vi "BRig_RT_panel_Laser2_v1,10.vi"(7 "input_setValues":bool, 9 "input_dataExp":u16[](array[numeric]), 11 "input_dataLC":u16[](array[numeric])) -> (1 "output_dataExp":u16[](array[numeric]), 3 "output_dataLC":u16[](array[numeric]))   [LabVIEW 2014]
panel:
  in  "LC_Cue2_PostR_Count":u16
  in  "LC_Cue2_PostR_delayOpt":bool
  in  "LC_Cue2_PostR_Probability":u16
  in  "LC_Cue2_PostR_Block":u16(slide) max=2 step=1 scale=0.0..2.0
  in  "LC_Cue2_PostR_OnOff":bool
  in  "LC_Cue2_PostR_Tdelay":u16
  in  "LC_ENL2_PostR_delayOpt":bool
  in  "LC_ENL2_PostR_Count":u16
  in  "LC_ENL2_PostR_Probability":u16 max=100 step=1
  in  "LC_ENL2_PostR_Block":u16(slide) max=2 step=1 scale=0.0..2.0
  in  "LC_ENL2_PostR_OnOff":bool
  in  "LC_ENL2_PostR_Tdelay":u16
  in  "LC_Cue2_PreR_Count":u16
  in  "LC_Cue2_First_Count":u16
  in  "LC_Cue2_PreR_delayOpt":bool
  in  "LC_ENL2_PreR_delayOpt":bool
  in  "LC_ENL2_PreR_Count":u16
  in  "LC_ENL2_First_Count":u16
  in  "LC_Cue2_First_delayOpt":bool
  in  "LC_ENL2_First_delayOpt":bool
  in  "LC_Cue2_PreR_Probability":u16
  in  "LC_Cue2_PreR_Block":u16(slide) max=2 step=1 scale=0.0..2.0
  in  "LC_Cue2_PreR_OnOff":bool
  in  "LC_Cue2_First_Probability":u16
  in  "LC_Cue2_First_Block":u16(slide) max=2 step=1 scale=0.0..2.0
  in  "LC_Cue2_First_OnOff":bool
  in  "LC_ENL2_PreR_Probability":u16 max=100 step=1
  in  "LC_ENL2_PreR_Block":u16(slide) max=2 step=1 scale=0.0..2.0
  in  "LC_ENL2_PreR_OnOff":bool
  in  "LC_ENL2_First_Probability":u16 max=100 step=1
  in  "LC_ENL2_First_Block":u16(slide) max=2 step=1 scale=0.0..2.0
  in  "LC_Cue2_PreR_Tdelay":u16
  in  "LC_ENL2_PreR_Tdelay":u16
  in  "LC_Cue2_First_Tdelay":u16
  in  "LC_ENL2_First_Tdelay":u16
  in  "LC_ENL2_First_OnOff":bool
  out "LaserPulseTrain":cluster{u16[], u16[]}(graph)
  in  "LED_baseline":bool
  in  "Laser_power_step":dbl
  in  "Laser_power_max":dbl
  in  "Laser_power_min":dbl
  in  "Laser_Tshutter":u16=2
  in  "Laser_Freq":u16=10
  in  "Laser_Tpeak":u16=2
  in  "Laser_T":u16
  in  "LC_Sel_PostR_Count":u16
  in  "LC_Sel_PostR_Probability":u16
  in  "LC_Sel_PostR_Block":u16(slide) max=2 step=1 scale=0.0..2.0
  in  "LC_Sel_PostR_OnOff":bool
  in  "LC_Sel_PostR_Tdelay":u16
  in  "LC_Cue_PostR_Count":u16
  in  "LC_Cue_PostR_delayOpt":bool
  in  "LC_Cue_PostR_Probability":u16
  in  "LC_Cue_PostR_Block":u16(slide) max=2 step=1 scale=0.0..2.0
  in  "LC_Cue_PostR_OnOff":bool
  in  "LC_Cue_PostR_Tdelay":u16
  in  "LC_ENL_PostR_delayOpt":bool
  in  "LC_ENL_PostR_Count":u16
  in  "LC_ENL_PostR_Probability":u16 max=100 step=1
  in  "LC_ENL_PostR_Block":u16(slide) max=2 step=1 scale=0.0..2.0
  in  "LC_ENL_PostR_OnOff":bool
  in  "LC_ENL_PostR_Tdelay":u16
  in  "LC_Sel_PreR_Count":u16
  in  "LC_Sel_First_Count":u16
  in  "LC_Sel_PreR_Probability":u16
  in  "LC_Sel_PreR_Block":u16(slide) max=2 step=1 scale=0.0..2.0
  in  "LC_Sel_PreR_OnOff":bool
  in  "LC_Sel_First_Probability":u16
  in  "LC_Sel_First_Block":u16(slide) max=2 step=1 scale=0.0..2.0
  in  "LC_Sel_First_OnOff":bool
  in  "LC_Sel_PreR_Tdelay":u16
  in  "LC_Sel_First_Tdelay":u16
  in  "LC_Cue_PreR_Count":u16
  in  "LC_Cue_First_Count":u16
  in  "LC_Cue_PreR_delayOpt":bool
  in  "LC_ENL_PreR_delayOpt":bool
  in  "LC_ENL_PreR_Count":u16
  in  "LC_ENL_First_Count":u16
  in  "LC_Cue_First_delayOpt":bool
  in  "LC_ENL_First_delayOpt":bool
  in  "LC_Wrong_Probability":u16
  in  "LC_Wrong_Trial":u16(slide) max=2 step=1 scale=0.0..2.0
  in  "LC_Wrong_Block":u16(slide) max=2 step=1 scale=0.0..2.0
  in  "LC_Wrong_OnOff":bool
  in  "LC_Reward_Probability":u16
  in  "LC_Reward_Trial":u16(slide) max=2 step=1 scale=0.0..2.0
  in  "LC_Reward_Block":u16(slide) max=2 step=1 scale=0.0..2.0
  in  "LC_Reward_OnOff":bool
  in  "LC_Cue_PreR_Probability":u16
  in  "LC_Cue_PreR_Block":u16(slide) max=2 step=1 scale=0.0..2.0
  in  "LC_Cue_PreR_OnOff":bool
  in  "LC_Cue_First_Probability":u16
  in  "LC_Cue_First_Block":u16(slide) max=2 step=1 scale=0.0..2.0
  in  "LC_Cue_First_OnOff":bool
  in  "LC_ENL_PreR_Probability":u16 max=100 step=1
  in  "LC_ENL_PreR_Block":u16(slide) max=2 step=1 scale=0.0..2.0
  in  "LC_ENL_PreR_OnOff":bool
  in  "LC_ENL_First_Probability":u16 max=100 step=1
  in  "LC_ENL_First_Block":u16(slide) max=2 step=1 scale=0.0..2.0
  in  "LC_Wrong_Tdelay":u16
  in  "LC_Cue_PreR_Tdelay":u16
  in  "LC_ENL_PreR_Tdelay":u16
  in  "LC_Reward_Tdelay":u16
  in  "LC_Cue_First_Tdelay":u16
  in  "LC_ENL_First_Tdelay":u16
  in  "LC_ENL_First_OnOff":bool
  # "Laser2 Control\n                               On/Off      Block        Probability [%]   Delay [ms]                              Count"
  # "On/Off      Block        Probability [%]   Delay [ms]                              Count"
  # "Enforced\nNonLick"
  # "Enforced\nNonLick\n     2"
  # "from end"
  # "from end"
  # "First\nTrial"
  # "First\nTrial"
  # "from start"
  # "from start"
  # "from end"
  # "from end"
  # "PreReward\nTrials"
  # "PreReward\nTrials"
  # "from start"
  # "from start"
  # "from end"
  # "from end"
  # "PostReward\nTrials"
  # "PostReward\nTrials"
  # "from start"
  # "from start"
  # "Cue"
  # "Cue\n  2"
  # "from end"
  # "from end"
  # "First\nTrial"
  # "First\nTrial"
  # "from start"
  # "from start"
  # "from end"
  # "from end"
  # "PreReward\nTrials"
  # "PreReward\nTrials"
  # "from start"
  # "from start"
  # "from end"
  # "from end"
  # "PostReward\nTrials"
  # "PostReward\nTrials"
  # "from start"
  # "from start"
  # "Selection"
  # "from start"
  # "First\nTrial"
  # "from start"
  # "PreReward\nTrials"
  # "from start"
  # "PostReward\nTrials"
  # "Laser2 Parameters"
  # "Laser2 Response\n           On/Off      Block           Trial     Probability %  Delay [ms]"
  # "Frequency\n[Hz]"
  # "Selection\nReward"
  # "Timing [ms]\n Duration     Peak Width   Shutter"
  # "Selection\nWrong"
  # "Laser Power [V]\nMin          Max              Step"
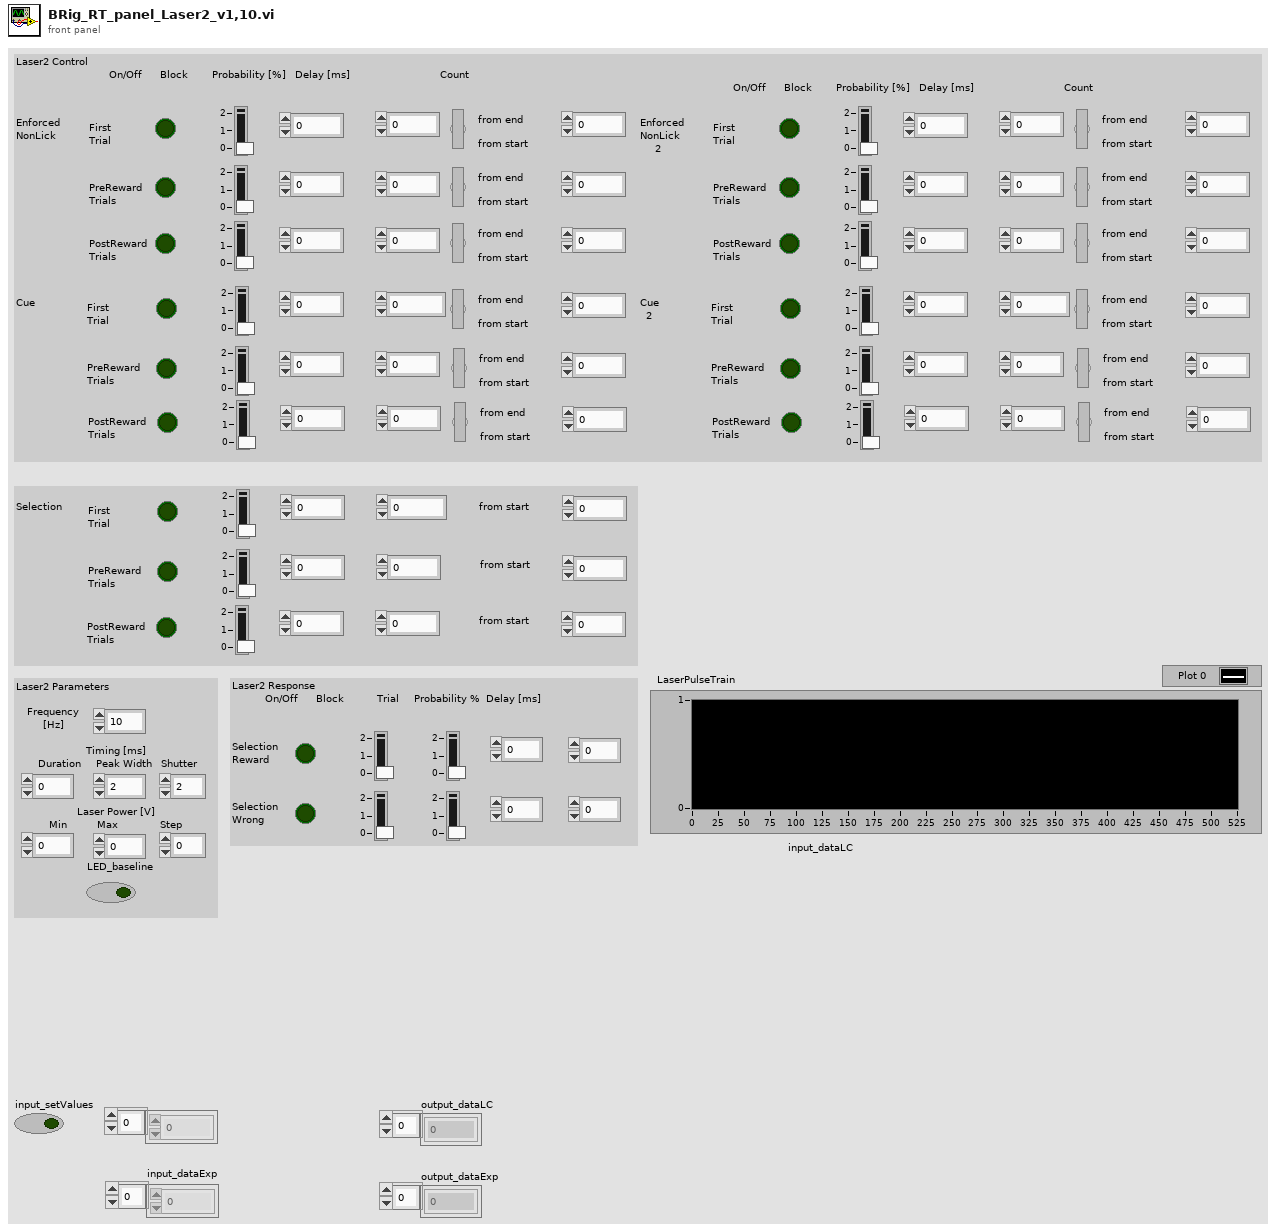
[diagram p1: front panel]
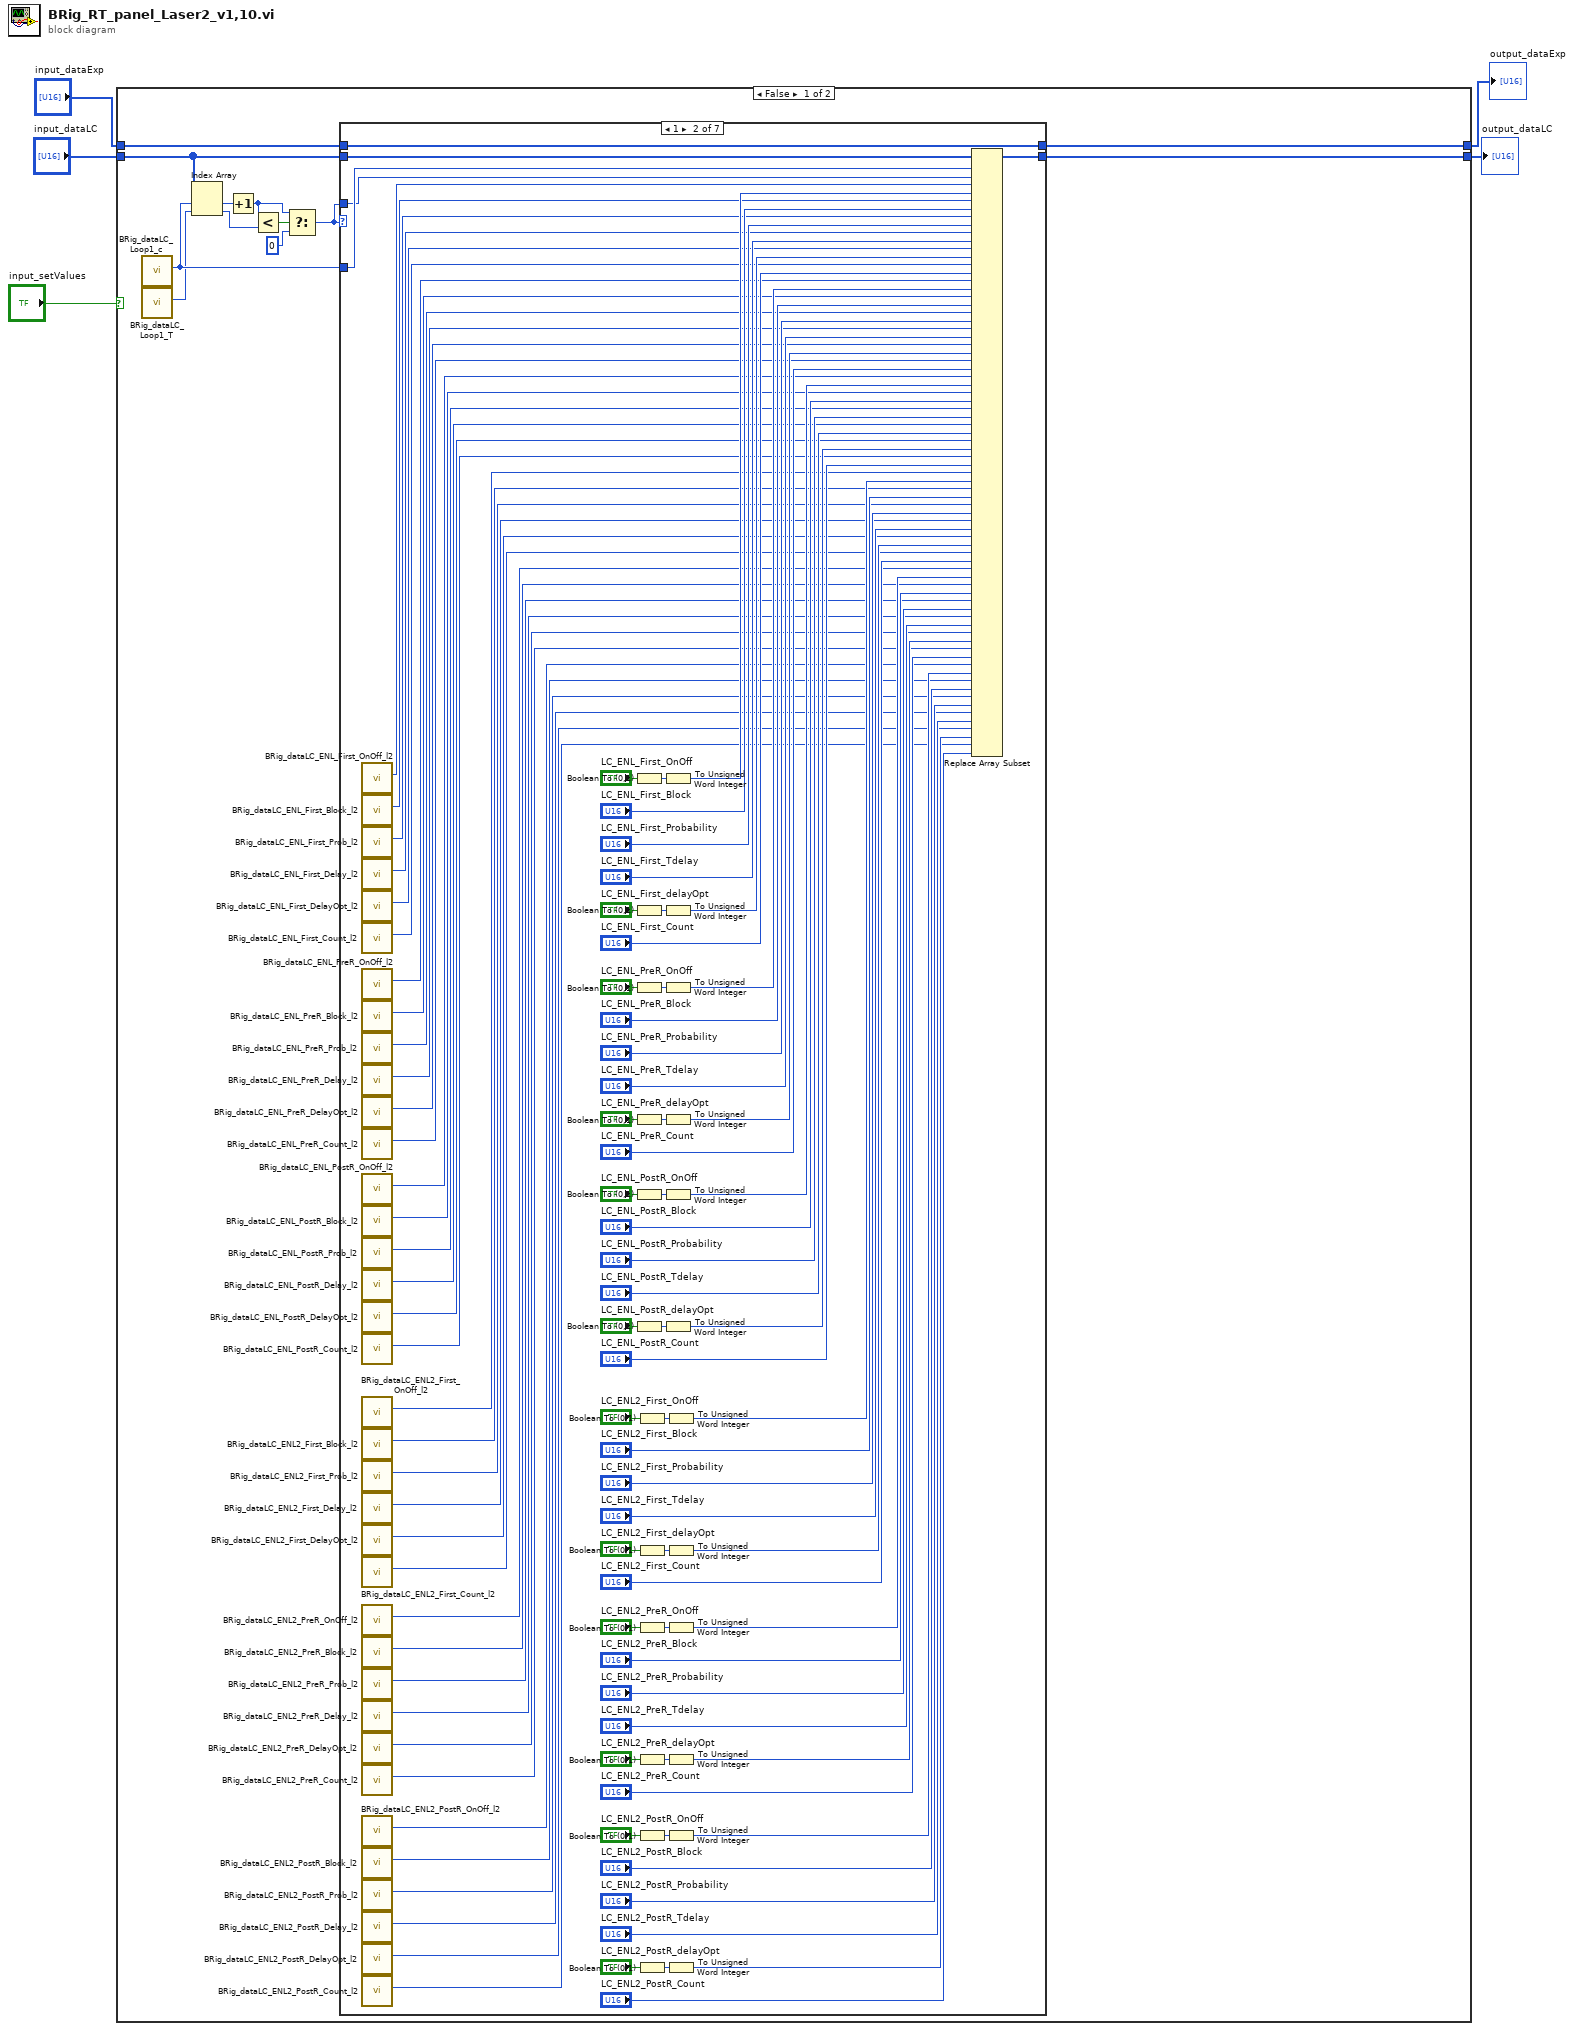
[diagram p0: block diagram]
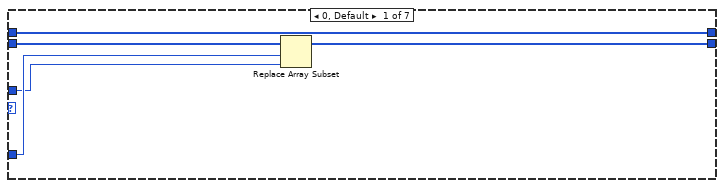
[diagram p2: hidden frame]
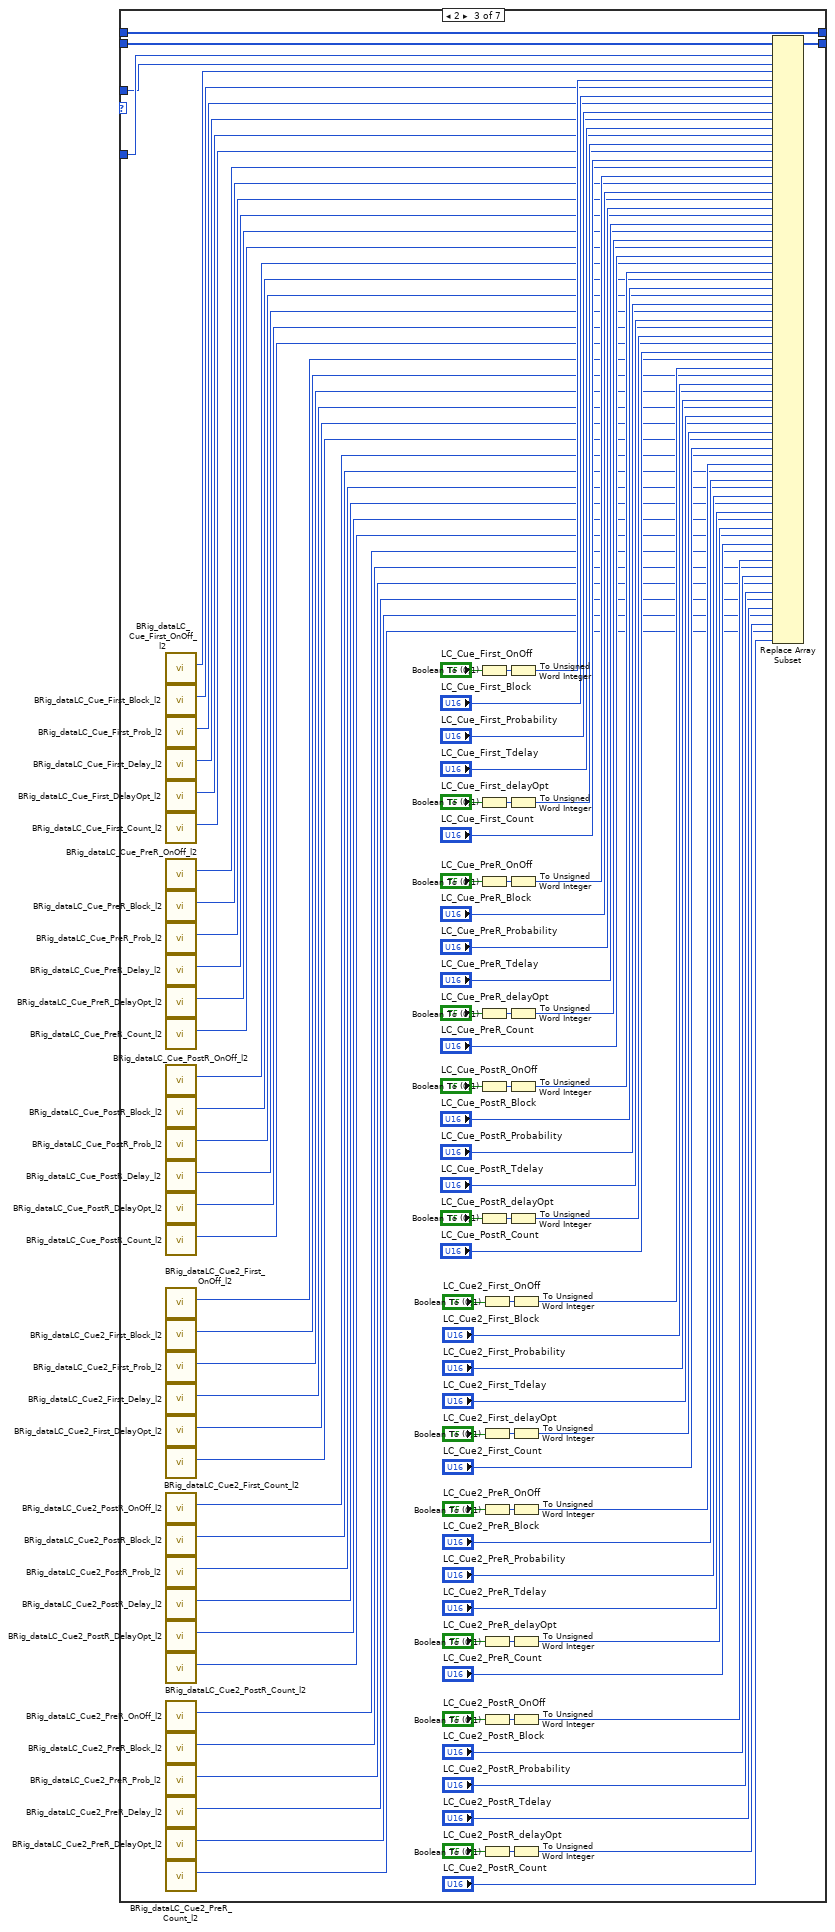
[diagram p3: hidden frame]
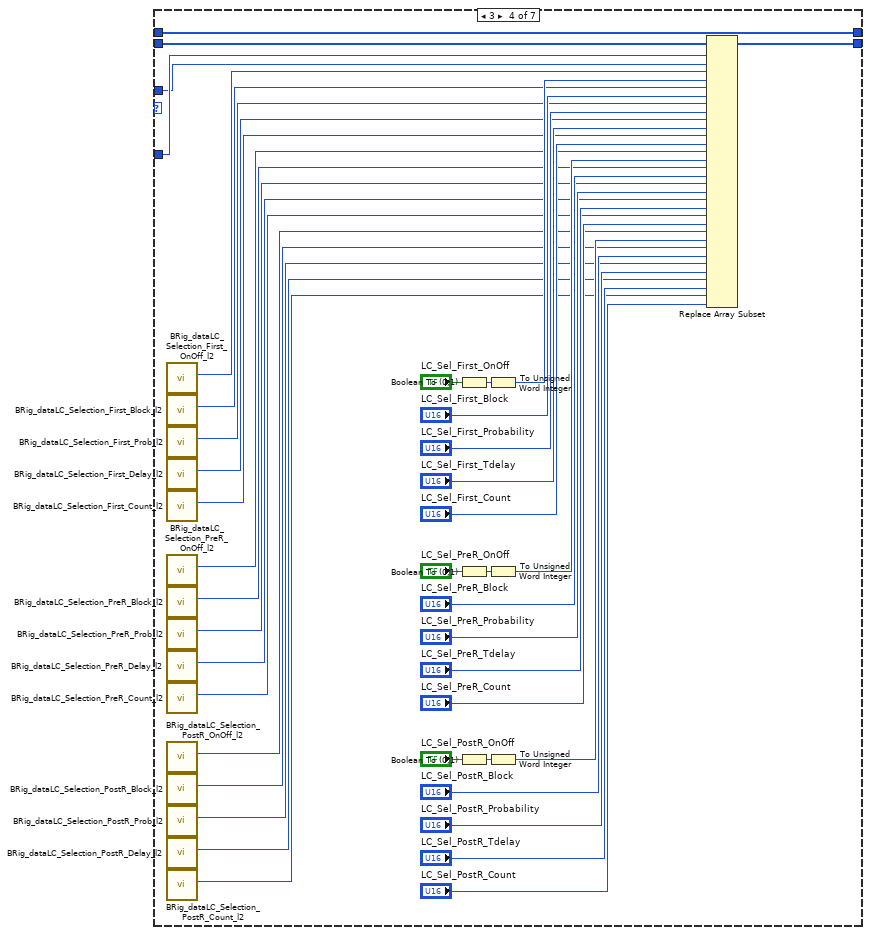
[diagram p4: hidden frame]
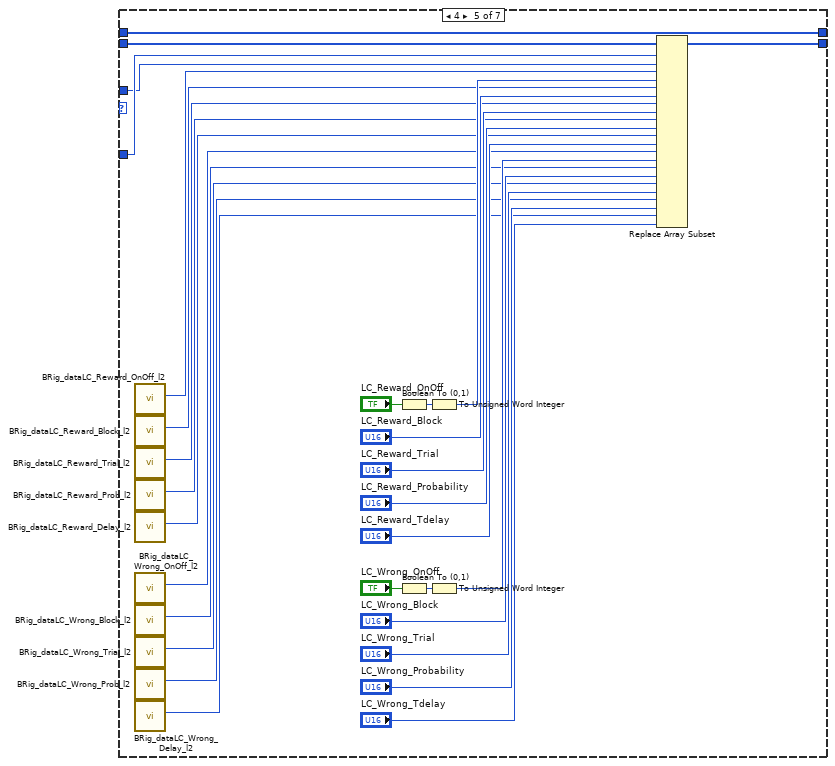
[diagram p5: hidden frame]
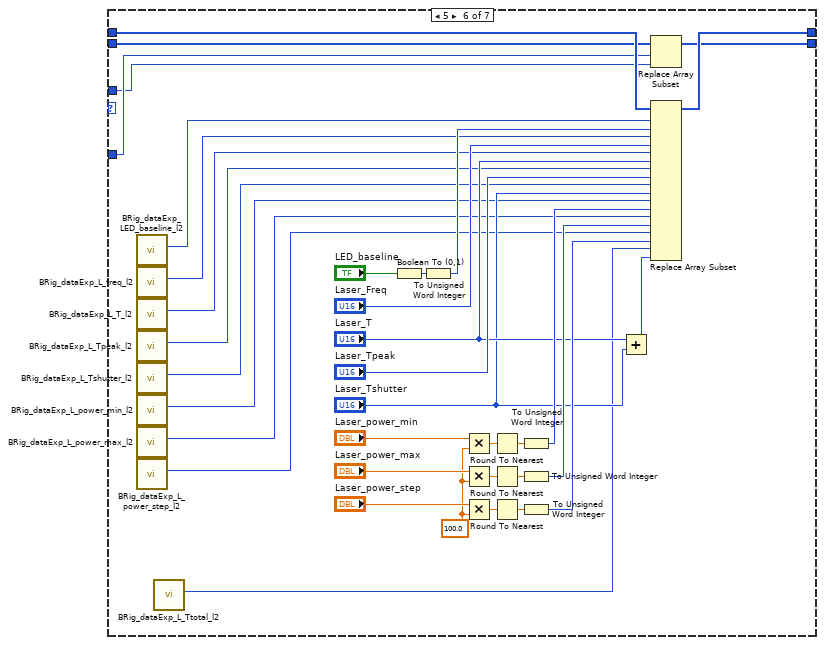
[diagram p6: hidden frame]
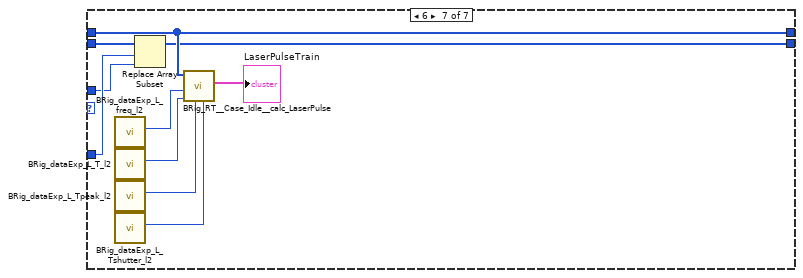
[diagram p7: hidden frame]
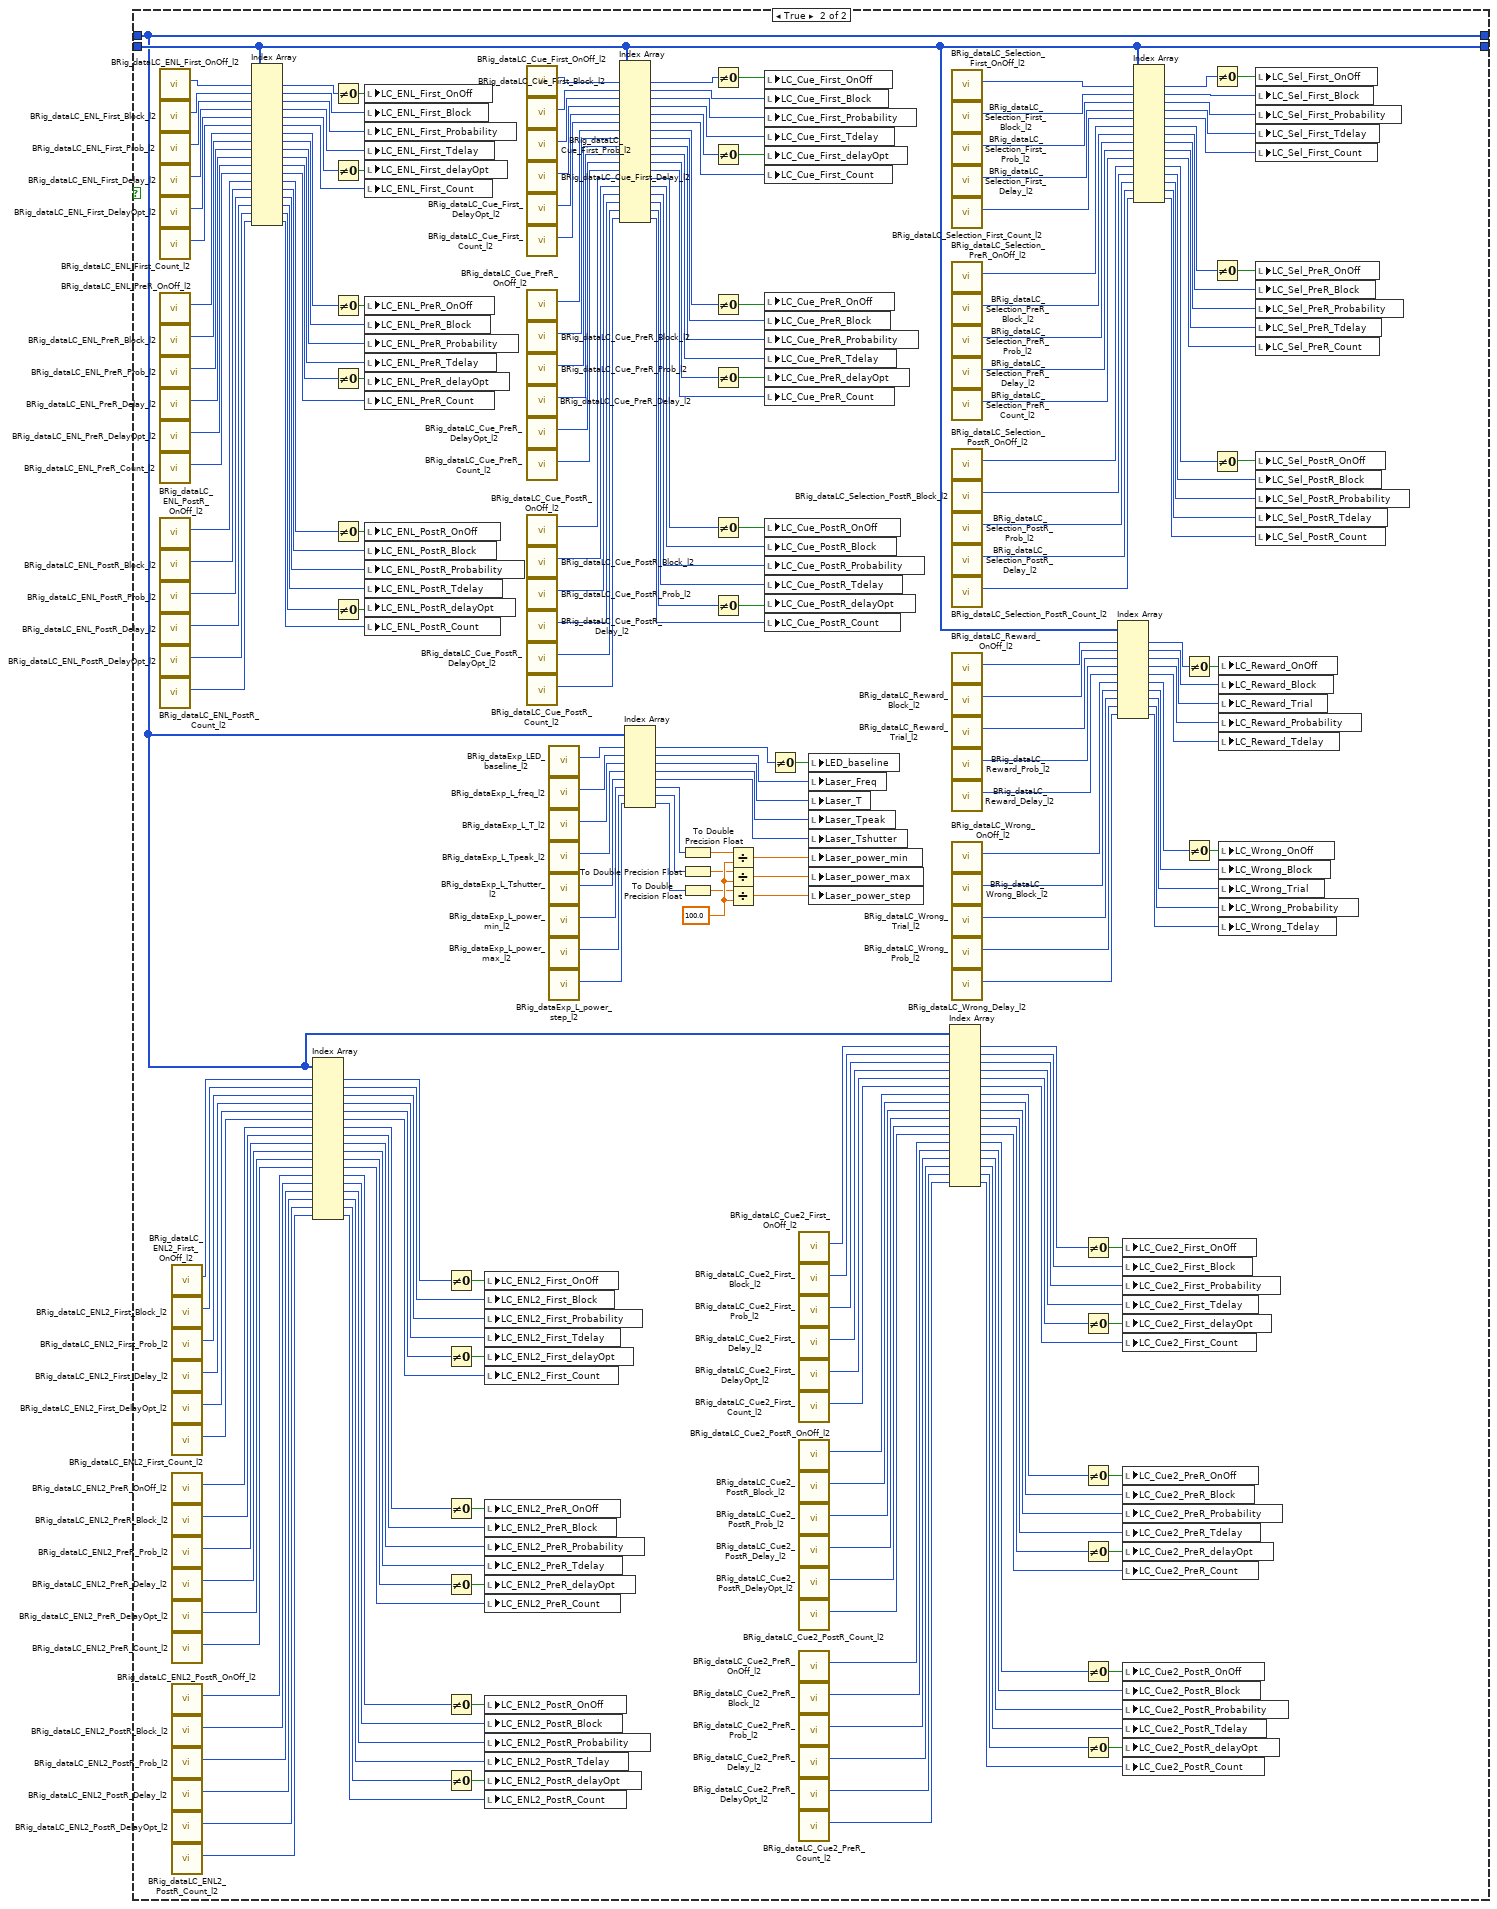
[diagram p8: hidden frame]
diagram:
  n1 = case shown="False" "input_setValues" {
    tunnel: "input_dataLC" -> [w17 w511]
    tunnel: [w11 w511] -> w4
    tunnel: "input_dataExp" -> [w7 w464]
    tunnel: [w6 w464] -> w1
    frame False {
      n2 = call "BRig_dataLC_Loop1_c.vi"() -> ("output_Loop1_c"=w10:i32)  [unwired: 11 in]
      n3 = call "BRig_dataLC_Loop1_T.vi"() -> ("output_Loop1_T"=w9:i32)  [unwired: 11 in]
      n4 = Index Array(array=w17, index #1=w10, index #2=w9) -> (element #1=w16:u16, element #2=w15:u16)
      n5 = Increment(x=w16) -> (x+1=w12:u16)
      n6 = Less?(x=w12, y=w15) -> (x < y?=w14:bool)
      n7 = Select(t=w12, s=w14, f=u16 0) -> (s? t:f=w8:u16)
      n8 = case shown="1" w8 {
        tunnel: w17 -> [w22 w123 w224 w265 w294 w307 w338]
        tunnel: w10 -> [w20 w91 w192 w242 w278 w305 w336]
        tunnel: w8 -> [w19 w90 w191 w241 w277 w304 w335]
        tunnel: [w21 w122 w223 w264 w293 w306 w337] -> w11
        tunnel: w7 -> [w18 w89 w190 w240 w276 w309 w340]
        tunnel: [w18 w89 w190 w240 w276 w308 w340] -> w6
        frame 0, Default {
          n9 = Replace Array Subset(array=w22, new element=w19, index=w20) -> (w21:u16[])
        }
        frame 1 {
          n10 = call "BRig_dataLC_ENL_First_OnOff_l2.vi"() -> ("output_ENL_First_OnOff_l2"=w41:i32)  [unwired: 11 in]
          n11 = call "BRig_dataLC_ENL_First_Block_l2.vi"() -> ("output_ENL_First_Block_l2"=w42:i32)  [unwired: 11 in]
          n12 = call "BRig_dataLC_ENL_First_Prob_l2.vi"() -> ("output_ENL_First_Prob_l2"=w43:i32)  [unwired: 11 in]
          n13 = call "BRig_dataLC_ENL_First_Delay_l2.vi"() -> ("output_ENL_First_Delay_l2"=w44:i32)  [unwired: 11 in]
          n14 = call "BRig_dataLC_ENL_First_DelayOpt_l2.vi"() -> ("output_ENL_First_DelayOpt_l2"=w45:i32)  [unwired: 11 in]
          n15 = call "BRig_dataLC_ENL_First_Count_l2.vi"() -> ("output_ENL_First_Count_l2"=w46:i32)  [unwired: 11 in]
          n16 = call "BRig_dataLC_ENL_PreR_OnOff_l2.vi"() -> ("output_ENL_PreR_OnOff_l2"=w47:i32)  [unwired: 11 in]
          n17 = call "BRig_dataLC_ENL_PreR_Block_l2.vi"() -> ("output_ENL_PreR_Block_l2"=w48:i32)  [unwired: 11 in]
          n18 = call "BRig_dataLC_ENL_PreR_Prob_l2.vi"() -> ("output_ENL_PreR_Prob_l2"=w49:i32)  [unwired: 11 in]
          n19 = call "BRig_dataLC_ENL_PreR_Delay_l2.vi"() -> ("output_ENL_PreR_Delay_l2"=w50:i32)  [unwired: 11 in]
          n20 = call "BRig_dataLC_ENL_PreR_DelayOpt_l2.vi"() -> ("output_ENL_PreR_DelayOpt_l2"=w51:i32)  [unwired: 11 in]
          n21 = call "BRig_dataLC_ENL_PreR_Count_l2.vi"() -> ("output_ENL_PreR_Count_l2"=w52:i32)  [unwired: 11 in]
          n22 = call "BRig_dataLC_ENL_PostR_OnOff_l2.vi"() -> ("output_ENL_PostR_OnOff_l2"=w53:i32)  [unwired: 11 in]
          n23 = call "BRig_dataLC_ENL_PostR_Block_l2.vi"() -> ("output_ENL_PostR_Block_l2"=w54:i32)  [unwired: 11 in]
          n24 = call "BRig_dataLC_ENL_PostR_Prob_l2.vi"() -> ("output_ENL_PostR_Prob_l2"=w55:i32)  [unwired: 11 in]
          n25 = call "BRig_dataLC_ENL_PostR_Delay_l2.vi"() -> ("output_ENL_PostR_Delay_l2"=w56:i32)  [unwired: 11 in]
          n26 = call "BRig_dataLC_ENL_PostR_DelayOpt_l2.vi"() -> ("output_ENL_PostR_DelayOpt_l2"=w57:i32)  [unwired: 11 in]
          n27 = call "BRig_dataLC_ENL_PostR_Count_l2.vi"() -> ("output_ENL_PostR_Count_l2"=w58:i32)  [unwired: 11 in]
          n28 = call "BRig_dataLC_ENL2_First_OnOff_l2.vi"() -> ("output_ENL2_First_OnOff_l2"=w40:i32)  [unwired: 11 in]
          n29 = call "BRig_dataLC_ENL2_First_Block_l2.vi"() -> ("output_ENL2_First_Block_l2"=w39:i32)  [unwired: 11 in]
          n30 = call "BRig_dataLC_ENL2_First_Prob_l2.vi"() -> ("output_ENL2_First_Prob_l2"=w38:i32)  [unwired: 11 in]
          n31 = call "BRig_dataLC_ENL2_First_Delay_l2.vi"() -> ("output_ENL2_First_Delay_l2"=w37:i32)  [unwired: 11 in]
          n32 = call "BRig_dataLC_ENL2_First_DelayOpt_l2.vi"() -> ("output_ENL2_First_DelayOpt_l2"=w36:i32)  [unwired: 11 in]
          n33 = call "BRig_dataLC_ENL2_First_Count_l2.vi"() -> ("output_ENL2_First_Count_l2"=w35:i32)  [unwired: 11 in]
          n34 = call "BRig_dataLC_ENL2_PreR_OnOff_l2.vi"() -> ("output_ENL2_PreR_OnOff_l2"=w34:i32)  [unwired: 11 in]
          n35 = call "BRig_dataLC_ENL2_PreR_Block_l2.vi"() -> ("output_ENL2_PreR_Block_l2"=w33:i32)  [unwired: 11 in]
          n36 = call "BRig_dataLC_ENL2_PreR_Prob_l2.vi"() -> ("output_ENL2_PreR_Prob_l2"=w32:i32)  [unwired: 11 in]
          n37 = call "BRig_dataLC_ENL2_PreR_Delay_l2.vi"() -> ("output_ENL2_PreR_Delay_l2"=w31:i32)  [unwired: 11 in]
          n38 = call "BRig_dataLC_ENL2_PreR_DelayOpt_l2.vi"() -> ("output_ENL2_PreR_DelayOpt_l2"=w30:i32)  [unwired: 11 in]
          n39 = call "BRig_dataLC_ENL2_PreR_Count_l2.vi"() -> ("output_ENL2_PreR_Count_l2"=w29:i32)  [unwired: 11 in]
          n40 = call "BRig_dataLC_ENL2_PostR_OnOff_l2.vi"() -> ("output_ENL2_PostR_OnOff_l2"=w28:i32)  [unwired: 11 in]
          n41 = call "BRig_dataLC_ENL2_PostR_Block_l2.vi"() -> ("output_ENL2_PostR_Block_l2"=w27:i32)  [unwired: 11 in]
          n42 = call "BRig_dataLC_ENL2_PostR_Prob_l2.vi"() -> ("output_ENL2_PostR_Prob_l2"=w26:i32)  [unwired: 11 in]
          n43 = call "BRig_dataLC_ENL2_PostR_Delay_l2.vi"() -> ("output_ENL2_PostR_Delay_l2"=w25:i32)  [unwired: 11 in]
          n44 = call "BRig_dataLC_ENL2_PostR_DelayOpt_l2.vi"() -> ("output_ENL2_PostR_DelayOpt_l2"=w24:i32)  [unwired: 11 in]
          n45 = call "BRig_dataLC_ENL2_PostR_Count_l2.vi"() -> ("output_ENL2_PostR_Count_l2"=w23:i32)  [unwired: 11 in]
          n46 = Boolean To (0,1)(Boolean="LC_ENL_First_OnOff") -> (0, 1=w120:i16)
          n47 = Boolean To (0,1)(Boolean="LC_ENL_First_delayOpt") -> (0, 1=w119:i16)
          n48 = Boolean To (0,1)(Boolean="LC_ENL_PreR_OnOff") -> (0, 1=w117:i16)
          n49 = Boolean To (0,1)(Boolean="LC_ENL_PreR_delayOpt") -> (0, 1=w115:i16)
          n50 = Boolean To (0,1)(Boolean="LC_ENL_PostR_OnOff") -> (0, 1=w113:i16)
          n51 = Boolean To (0,1)(Boolean="LC_ENL_PostR_delayOpt") -> (0, 1=w111:i16)
          n52 = Boolean To (0,1)(Boolean="LC_ENL2_First_OnOff") -> (0, 1=w79:i16)
          n53 = Boolean To (0,1)(Boolean="LC_ENL2_First_delayOpt") -> (0, 1=w78:i16)
          n54 = Boolean To (0,1)(Boolean="LC_ENL2_PreR_OnOff") -> (0, 1=w77:i16)
          n55 = Boolean To (0,1)(Boolean="LC_ENL2_PreR_delayOpt") -> (0, 1=w75:i16)
          n56 = Boolean To (0,1)(Boolean="LC_ENL2_PostR_OnOff") -> (0, 1=w67:i16)
          n57 = Boolean To (0,1)(Boolean="LC_ENL2_PostR_delayOpt") -> (0, 1=w65:i16)
          n58 = To Unsigned Word Integer(number=w120) -> (unsigned 16bit integer=w109:u16)
          n59 = To Unsigned Word Integer(number=w119) -> (unsigned 16bit integer=w105:u16)
          n60 = To Unsigned Word Integer(number=w117) -> (unsigned 16bit integer=w103:u16)
          n61 = To Unsigned Word Integer(number=w115) -> (unsigned 16bit integer=w99:u16)
          n62 = To Unsigned Word Integer(number=w113) -> (unsigned 16bit integer=w97:u16)
          n63 = To Unsigned Word Integer(number=w111) -> (unsigned 16bit integer=w93:u16)
          n64 = To Unsigned Word Integer(number=w79) -> (unsigned 16bit integer=w86:u16)
          n65 = To Unsigned Word Integer(number=w78) -> (unsigned 16bit integer=w82:u16)
          n66 = To Unsigned Word Integer(number=w77) -> (unsigned 16bit integer=w80:u16)
          n67 = To Unsigned Word Integer(number=w75) -> (unsigned 16bit integer=w70:u16)
          n68 = To Unsigned Word Integer(number=w67) -> (unsigned 16bit integer=w68:u16)
          n69 = To Unsigned Word Integer(number=w65) -> (unsigned 16bit integer=w60:u16)
          n70 = Replace Array Subset(array=w123, new element #1=w90, index #1=w91, new element #2=w109, index #2=w41, new element #3="LC_ENL_First_Block", index #3=w42, new element #4="LC_ENL_First_Probability", index #4=w43, new element #5="LC_ENL_First_Tdelay", index #5=w44, new element #6=w105, index #6=w45, new element #7="LC_ENL_First_Count", index #7=w46, new element #8=w103, index #8=w47, new element #9="LC_ENL_PreR_Block", index #9=w48, new element #10="LC_ENL_PreR_Probability", index #10=w49, new element #11="LC_ENL_PreR_Tdelay", index #11=w50, new element #12=w99, index #12=w51, new element #13="LC_ENL_PreR_Count", index #13=w52, new element #14=w97, index #14=w53, new element #15="LC_ENL_PostR_Block", index #15=w54, new element #16="LC_ENL_PostR_Probability", index #16=w55, new element #17="LC_ENL_PostR_Tdelay", index #17=w56, new element #18=w93, index #18=w57, new element #19="LC_ENL_PostR_Count", index #19=w58, new element #20=w86, index #20=w40, new element #21="LC_ENL2_First_Block", index #21=w39, new element #22="LC_ENL2_First_Probability", index #22=w38, new element #23="LC_ENL2_First_Tdelay", index #23=w37, new element #24=w82, index #24=w36, new element #25="LC_ENL2_First_Count", index #25=w35, new element #26=w80, index #26=w34, new element #27="LC_ENL2_PreR_Block", index #27=w33, new element #28="LC_ENL2_PreR_Probability", index #28=w32, new element #29="LC_ENL2_PreR_Tdelay", index #29=w31, new element #30=w70, index #30=w30, new element #31="LC_ENL2_PreR_Count", index #31=w29, new element #32=w68, index #32=w28, new element #33="LC_ENL2_PostR_Block", index #33=w27, new element #34="LC_ENL2_PostR_Probability", index #34=w26, new element #35="LC_ENL2_PostR_Tdelay", index #35=w25, new element #36=w60, index #36=w24, new element #37="LC_ENL2_PostR_Count", index #37=w23) -> (w122:u16[])
        }
        frame 2 {
          n71 = call "BRig_dataLC_Cue_First_OnOff_l2.vi"() -> ("output_Cue_First_OnOff_l2"=w142:i32)  [unwired: 11 in]
          n72 = call "BRig_dataLC_Cue_First_Block_l2.vi"() -> ("output_Cue_First_Block_l2"=w143:i32)  [unwired: 11 in]
          n73 = call "BRig_dataLC_Cue_First_Prob_l2.vi"() -> ("output_Cue_First_Prob_l2"=w144:i32)  [unwired: 11 in]
          n74 = call "BRig_dataLC_Cue_First_Delay_l2.vi"() -> ("output_Cue_First_Delay_l2"=w145:i32)  [unwired: 11 in]
          n75 = call "BRig_dataLC_Cue_First_DelayOpt_l2.vi"() -> ("output_Cue_First_DelayOpt_l2"=w146:i32)  [unwired: 11 in]
          n76 = call "BRig_dataLC_Cue_First_Count_l2.vi"() -> ("output_Cue_First_Count_l2"=w147:i32)  [unwired: 11 in]
          n77 = call "BRig_dataLC_Cue_PreR_OnOff_l2.vi"() -> ("output_Cue_PreR_OnOff_l2"=w148:i32)  [unwired: 11 in]
          n78 = call "BRig_dataLC_Cue_PreR_Block_l2.vi"() -> ("output_Cue_PreR_Block_l2"=w149:i32)  [unwired: 11 in]
          n79 = call "BRig_dataLC_Cue_PreR_Prob_l2.vi"() -> ("output_Cue_PreR_Prob_l2"=w150:i32)  [unwired: 11 in]
          n80 = call "BRig_dataLC_Cue_PreR_Delay_l2.vi"() -> ("output_Cue_PreR_Delay_l2"=w151:i32)  [unwired: 11 in]
          n81 = call "BRig_dataLC_Cue_PreR_DelayOpt_l2.vi"() -> ("output_Cue_PreR_DelayOpt_l2"=w152:i32)  [unwired: 11 in]
          n82 = call "BRig_dataLC_Cue_PreR_Count_l2.vi"() -> ("output_Cue_PreR_Count_l2"=w153:i32)  [unwired: 11 in]
          n83 = call "BRig_dataLC_Cue_PostR_OnOff_l2.vi"() -> ("output_Cue_PostR_OnOff_l2"=w154:i32)  [unwired: 11 in]
          n84 = call "BRig_dataLC_Cue_PostR_Block_l2.vi"() -> ("output_Cue_PostR_Block_l2"=w155:i32)  [unwired: 11 in]
          n85 = call "BRig_dataLC_Cue_PostR_Prob_l2.vi"() -> ("output_Cue_PostR_Prob_l2"=w156:i32)  [unwired: 11 in]
          n86 = call "BRig_dataLC_Cue_PostR_Delay_l2.vi"() -> ("output_Cue_PostR_Delay_l2"=w157:i32)  [unwired: 11 in]
          n87 = call "BRig_dataLC_Cue_PostR_DelayOpt_l2.vi"() -> ("output_Cue_PostR_DelayOpt_l2"=w158:i32)  [unwired: 11 in]
          n88 = call "BRig_dataLC_Cue_PostR_Count_l2.vi"() -> ("output_Cue_PostR_Count_l2"=w159:i32)  [unwired: 11 in]
          n89 = call "BRig_dataLC_Cue2_First_OnOff_l2.vi"() -> ("output_Cue2_First_OnOff_l2"=w141:i32)  [unwired: 11 in]
          n90 = call "BRig_dataLC_Cue2_First_Block_l2.vi"() -> ("output_Cue2_First_Block_l2"=w140:i32)  [unwired: 11 in]
          n91 = call "BRig_dataLC_Cue2_First_Prob_l2.vi"() -> ("output_Cue2_First_Prob_l2"=w139:i32)  [unwired: 11 in]
          n92 = call "BRig_dataLC_Cue2_First_Delay_l2.vi"() -> ("output_Cue2_First_Delay_l2"=w138:i32)  [unwired: 11 in]
          n93 = call "BRig_dataLC_Cue2_First_DelayOpt_l2.vi"() -> ("output_Cue2_First_DelayOpt_l2"=w137:i32)  [unwired: 11 in]
          n94 = call "BRig_dataLC_Cue2_First_Count_l2.vi"() -> ("output_Cue2_First_Count_l2"=w136:i32)  [unwired: 11 in]
          n95 = call "BRig_dataLC_Cue2_PostR_OnOff_l2.vi"() -> ("output_Cue2_PostR_OnOff_l2"=w135:i32)  [unwired: 11 in]
          n96 = call "BRig_dataLC_Cue2_PostR_Block_l2.vi"() -> ("output_Cue2_PostR_Block_l2"=w134:i32)  [unwired: 11 in]
          n97 = call "BRig_dataLC_Cue2_PostR_Prob_l2.vi"() -> ("output_Cue2_PostR_Prob_l2"=w133:i32)  [unwired: 11 in]
          n98 = call "BRig_dataLC_Cue2_PostR_Delay_l2.vi"() -> ("output_Cue2_PostR_Delay_l2"=w132:i32)  [unwired: 11 in]
          n99 = call "BRig_dataLC_Cue2_PostR_DelayOpt_l2.vi"() -> ("output_Cue2_PostR_DelayOpt_l2"=w131:i32)  [unwired: 11 in]
          n100 = call "BRig_dataLC_Cue2_PostR_Count_l2.vi"() -> ("output_Cue2_PostR_Count_l2"=w130:i32)  [unwired: 11 in]
          n101 = call "BRig_dataLC_Cue2_PreR_OnOff_l2.vi"() -> ("output_Cue2_PreR_OnOff_l2"=w129:i32)  [unwired: 11 in]
          n102 = call "BRig_dataLC_Cue2_PreR_Block_l2.vi"() -> ("output_Cue2_PreR_Block_l2"=w128:i32)  [unwired: 11 in]
          n103 = call "BRig_dataLC_Cue2_PreR_Prob_l2.vi"() -> ("output_Cue2_PreR_Prob_l2"=w127:i32)  [unwired: 11 in]
          n104 = call "BRig_dataLC_Cue2_PreR_Delay_l2.vi"() -> ("output_Cue2_PreR_Delay_l2"=w126:i32)  [unwired: 11 in]
          n105 = call "BRig_dataLC_Cue2_PreR_DelayOpt_l2.vi"() -> ("output_Cue2_PreR_DelayOpt_l2"=w125:i32)  [unwired: 11 in]
          n106 = call "BRig_dataLC_Cue2_PreR_Count_l2.vi"() -> ("output_Cue2_PreR_Count_l2"=w124:i32)  [unwired: 11 in]
          n107 = Boolean To (0,1)(Boolean="LC_Cue_First_OnOff") -> (0, 1=w216:i16)
          n108 = Boolean To (0,1)(Boolean="LC_Cue_First_delayOpt") -> (0, 1=w215:i16)
          n109 = Boolean To (0,1)(Boolean="LC_Cue_PreR_OnOff") -> (0, 1=w214:i16)
          n110 = Boolean To (0,1)(Boolean="LC_Cue_PreR_delayOpt") -> (0, 1=w213:i16)
          n111 = Boolean To (0,1)(Boolean="LC_Cue_PostR_OnOff") -> (0, 1=w212:i16)
          n112 = Boolean To (0,1)(Boolean="LC_Cue_PostR_delayOpt") -> (0, 1=w211:i16)
          n113 = Boolean To (0,1)(Boolean="LC_Cue2_First_OnOff") -> (0, 1=w189:i16)
          n114 = Boolean To (0,1)(Boolean="LC_Cue2_First_delayOpt") -> (0, 1=w188:i16)
          n115 = Boolean To (0,1)(Boolean="LC_Cue2_PreR_OnOff") -> (0, 1=w187:i16)
          n116 = Boolean To (0,1)(Boolean="LC_Cue2_PreR_delayOpt") -> (0, 1=w186:i16)
          n117 = Boolean To (0,1)(Boolean="LC_Cue2_PostR_OnOff") -> (0, 1=w185:i16)
          n118 = Boolean To (0,1)(Boolean="LC_Cue2_PostR_delayOpt") -> (0, 1=w184:i16)
          n119 = To Unsigned Word Integer(number=w216) -> (unsigned 16bit integer=w210:u16)
          n120 = To Unsigned Word Integer(number=w215) -> (unsigned 16bit integer=w206:u16)
          n121 = To Unsigned Word Integer(number=w214) -> (unsigned 16bit integer=w204:u16)
          n122 = To Unsigned Word Integer(number=w213) -> (unsigned 16bit integer=w200:u16)
          n123 = To Unsigned Word Integer(number=w212) -> (unsigned 16bit integer=w198:u16)
          n124 = To Unsigned Word Integer(number=w211) -> (unsigned 16bit integer=w194:u16)
          n125 = To Unsigned Word Integer(number=w189) -> (unsigned 16bit integer=w177:u16)
          n126 = To Unsigned Word Integer(number=w188) -> (unsigned 16bit integer=w173:u16)
          n127 = To Unsigned Word Integer(number=w187) -> (unsigned 16bit integer=w171:u16)
          n128 = To Unsigned Word Integer(number=w186) -> (unsigned 16bit integer=w167:u16)
          n129 = To Unsigned Word Integer(number=w185) -> (unsigned 16bit integer=w165:u16)
          n130 = To Unsigned Word Integer(number=w184) -> (unsigned 16bit integer=w161:u16)
          n131 = Replace Array Subset(array=w224, new element #1=w191, index #1=w192, new element #2=w210, index #2=w142, new element #3="LC_Cue_First_Block", index #3=w143, new element #4="LC_Cue_First_Probability", index #4=w144, new element #5="LC_Cue_First_Tdelay", index #5=w145, new element #6=w206, index #6=w146, new element #7="LC_Cue_First_Count", index #7=w147, new element #8=w204, index #8=w148, new element #9="LC_Cue_PreR_Block", index #9=w149, new element #10="LC_Cue_PreR_Probability", index #10=w150, new element #11="LC_Cue_PreR_Tdelay", index #11=w151, new element #12=w200, index #12=w152, new element #13="LC_Cue_PreR_Count", index #13=w153, new element #14=w198, index #14=w154, new element #15="LC_Cue_PostR_Block", index #15=w155, new element #16="LC_Cue_PostR_Probability", index #16=w156, new element #17="LC_Cue_PostR_Tdelay", index #17=w157, new element #18=w194, index #18=w158, new element #19="LC_Cue_PostR_Count", index #19=w159, new element #20=w177, index #20=w141, new element #21="LC_Cue2_First_Block", index #21=w140, new element #22="LC_Cue2_First_Probability", index #22=w139, new element #23="LC_Cue2_First_Tdelay", index #23=w138, new element #24=w173, index #24=w137, new element #25="LC_Cue2_First_Count", index #25=w136, new element #26=w171, index #26=w135, new element #27="LC_Cue2_PreR_Block", index #27=w134, new element #28="LC_Cue2_PreR_Probability", index #28=w133, new element #29="LC_Cue2_PreR_Tdelay", index #29=w132, new element #30=w167, index #30=w131, new element #31="LC_Cue2_PreR_Count", index #31=w130, new element #32=w165, index #32=w129, new element #33="LC_Cue2_PostR_Block", index #33=w128, new element #34="LC_Cue2_PostR_Probability", index #34=w127, new element #35="LC_Cue2_PostR_Tdelay", index #35=w126, new element #36=w161, index #36=w125, new element #37="LC_Cue2_PostR_Count", index #37=w124) -> (w223:u16[])
        }
        frame 3 {
          n132 = call "BRig_dataLC_Selection_First_OnOff_l2.vi"() -> ("output_Selection_First_OnOff_l2"=w225:i32)  [unwired: 11 in]
          n133 = call "BRig_dataLC_Selection_First_Block_l2.vi"() -> ("output_Selection_First_Block_l2"=w226:i32)  [unwired: 11 in]
          n134 = call "BRig_dataLC_Selection_First_Prob_l2.vi"() -> ("output_Selection_First_Prob_l2"=w227:i32)  [unwired: 11 in]
          n135 = call "BRig_dataLC_Selection_First_Delay_l2.vi"() -> ("output_Selection_First_Delay_l2"=w228:i32)  [unwired: 11 in]
          n136 = call "BRig_dataLC_Selection_First_Count_l2.vi"() -> ("output_Selection_First_Count_l2"=w229:i32)  [unwired: 11 in]
          n137 = call "BRig_dataLC_Selection_PreR_OnOff_l2.vi"() -> ("output_Selection_PreR_OnOff_l2"=w230:i32)  [unwired: 11 in]
          n138 = call "BRig_dataLC_Selection_PreR_Block_l2.vi"() -> ("output_Selection_PreR_Block_l2"=w231:i32)  [unwired: 11 in]
          n139 = call "BRig_dataLC_Selection_PreR_Prob_l2.vi"() -> ("output_Selection_PreR_Prob_l2"=w232:i32)  [unwired: 11 in]
          n140 = call "BRig_dataLC_Selection_PreR_Delay_l2.vi"() -> ("output_Selection_PreR_Delay_l2"=w233:i32)  [unwired: 11 in]
          n141 = call "BRig_dataLC_Selection_PreR_Count_l2.vi"() -> ("output_Selection_PreR_Count_l2"=w234:i32)  [unwired: 11 in]
          n142 = call "BRig_dataLC_Selection_PostR_OnOff_l2.vi"() -> ("output_Selection_PostR_OnOff_l2"=w235:i32)  [unwired: 11 in]
          n143 = call "BRig_dataLC_Selection_PostR_Block_l2.vi"() -> ("output_Selection_PostR_Block_l2"=w236:i32)  [unwired: 11 in]
          n144 = call "BRig_dataLC_Selection_PostR_Prob_l2.vi"() -> ("output_Selection_PostR_Prob_l2"=w237:i32)  [unwired: 11 in]
          n145 = call "BRig_dataLC_Selection_PostR_Delay_l2.vi"() -> ("output_Selection_PostR_Delay_l2"=w238:i32)  [unwired: 11 in]
          n146 = call "BRig_dataLC_Selection_PostR_Count_l2.vi"() -> ("output_Selection_PostR_Count_l2"=w239:i32)  [unwired: 11 in]
          n147 = Boolean To (0,1)(Boolean="LC_Sel_First_OnOff") -> (0, 1=w260:i16)
          n148 = Boolean To (0,1)(Boolean="LC_Sel_PreR_OnOff") -> (0, 1=w259:i16)
          n149 = Boolean To (0,1)(Boolean="LC_Sel_PostR_OnOff") -> (0, 1=w258:i16)
          n150 = To Unsigned Word Integer(number=w260) -> (unsigned 16bit integer=w257:u16)
          n151 = To Unsigned Word Integer(number=w259) -> (unsigned 16bit integer=w252:u16)
          n152 = To Unsigned Word Integer(number=w258) -> (unsigned 16bit integer=w247:u16)
          n153 = Replace Array Subset(array=w265, new element #1=w241, index #1=w242, new element #2=w257, index #2=w225, new element #3="LC_Sel_First_Block", index #3=w226, new element #4="LC_Sel_First_Probability", index #4=w227, new element #5="LC_Sel_First_Tdelay", index #5=w228, new element #6="LC_Sel_First_Count", index #6=w229, new element #7=w252, index #7=w230, new element #8="LC_Sel_PreR_Block", index #8=w231, new element #9="LC_Sel_PreR_Probability", index #9=w232, new element #10="LC_Sel_PreR_Tdelay", index #10=w233, new element #11="LC_Sel_PreR_Count", index #11=w234, new element #12=w247, index #12=w235, new element #13="LC_Sel_PostR_Block", index #13=w236, new element #14="LC_Sel_PostR_Probability", index #14=w237, new element #15="LC_Sel_PostR_Tdelay", index #15=w238, new element #16="LC_Sel_PostR_Count", index #16=w239) -> (w264:u16[])
        }
        frame 4 {
          n154 = call "BRig_dataLC_Reward_OnOff_l2.vi"() -> ("output_Reward_OnOff_l2"=w266:i32)  [unwired: 11 in]
          n155 = call "BRig_dataLC_Reward_Block_l2.vi"() -> ("output_Reward_Block_l2"=w267:i32)  [unwired: 11 in]
          n156 = call "BRig_dataLC_Reward_Trial_l2.vi"() -> ("output_Reward_Trial_l2"=w268:i32)  [unwired: 11 in]
          n157 = call "BRig_dataLC_Reward_Prob_l2.vi"() -> ("output_Reward_Prob_l2"=w269:i32)  [unwired: 11 in]
          n158 = call "BRig_dataLC_Reward_Delay_l2.vi"() -> ("output_Reward_Delay_l2"=w270:i32)  [unwired: 11 in]
          n159 = call "BRig_dataLC_Wrong_OnOff_l2.vi"() -> ("output_Wrong_OnOff_l2"=w271:i32)  [unwired: 11 in]
          n160 = call "BRig_dataLC_Wrong_Block_l2.vi"() -> ("output_Wrong_Block_l2"=w272:i32)  [unwired: 11 in]
          n161 = call "BRig_dataLC_Wrong_Trial_l2.vi"() -> ("output_Wrong_Trial_l2"=w273:i32)  [unwired: 11 in]
          n162 = call "BRig_dataLC_Wrong_Prob_l2.vi"() -> ("output_Wrong_Prob_l2"=w274:i32)  [unwired: 11 in]
          n163 = call "BRig_dataLC_Wrong_Delay_l2.vi"() -> ("output_Wrong_Delay_l2"=w275:i32)  [unwired: 11 in]
          n164 = Boolean To (0,1)(Boolean="LC_Reward_OnOff") -> (0, 1=w290:i16)
          n165 = Boolean To (0,1)(Boolean="LC_Wrong_OnOff") -> (0, 1=w289:i16)
          n166 = To Unsigned Word Integer(number=w290) -> (unsigned 16bit integer=w288:u16)
          n167 = To Unsigned Word Integer(number=w289) -> (unsigned 16bit integer=w283:u16)
          n168 = Replace Array Subset(array=w294, new element #1=w277, index #1=w278, new element #2=w288, index #2=w266, new element #3="LC_Reward_Block", index #3=w267, new element #4="LC_Reward_Trial", index #4=w268, new element #5="LC_Reward_Probability", index #5=w269, new element #6="LC_Reward_Tdelay", index #6=w270, new element #7=w283, index #7=w271, new element #8="LC_Wrong_Block", index #8=w272, new element #9="LC_Wrong_Trial", index #9=w273, new element #10="LC_Wrong_Probability", index #10=w274, new element #11="LC_Wrong_Tdelay", index #11=w275) -> (w293:u16[])
        }
        frame 5 {
          w318 = 100.0 ("y")
          n169 = call "BRig_dataExp_LED_baseline_l2.vi"() -> ("output_LED_baseline_l2"=w295:i32)  [unwired: 11 in]
          n170 = call "BRig_dataExp_L_freq_l2.vi"() -> ("output_L_freq_l2"=w296:i32)  [unwired: 11 in]
          n171 = call "BRig_dataExp_L_T_l2.vi"() -> ("output_L_T_l2"=w297:i32)  [unwired: 11 in]
          n172 = call "BRig_dataExp_L_Tpeak_l2.vi"() -> ("output_L_Tpeak_l2"=w298:i32)  [unwired: 11 in]
          n173 = call "BRig_dataExp_L_Tshutter_l2.vi"() -> ("output_L_Tshutter_l2"=w299:i32)  [unwired: 11 in]
          n174 = call "BRig_dataExp_L_power_min_l2.vi"() -> ("output_L_power_min_l2"=w300:i32)  [unwired: 11 in]
          n175 = call "BRig_dataExp_L_power_max_l2.vi"() -> ("output_L_power_max_l2"=w301:i32)  [unwired: 11 in]
          n176 = call "BRig_dataExp_L_power_step_l2.vi"() -> ("output_L_power_step_l2"=w302:i32)  [unwired: 11 in]
          n177 = call "BRig_dataExp_L_Ttotal_l2.vi"() -> ("output_L_Ttotal_l2"=w303:i32)  [unwired: 11 in]
          n178 = Boolean To (0,1)(Boolean="LED_baseline") -> (0, 1=w330:i16)
          n179 = To Unsigned Word Integer(number=w330) -> (unsigned 16bit integer=w328:u16)
          n180 = Multiply(x="Laser_power_min", y=w318) -> (x*y=w322:dbl)
          n181 = Multiply(x="Laser_power_max", y=w318) -> (x*y=w324:dbl)
          n182 = Multiply(x="Laser_power_step", y=w318) -> (x*y=w327:dbl)
          n183 = Round To Nearest(number=w322) -> (nearest integer value=w321:dbl)
          n184 = Round To Nearest(number=w324) -> (nearest integer value=w323:dbl)
          n185 = Round To Nearest(number=w327) -> (nearest integer value=w326:dbl)
          n186 = To Unsigned Word Integer(number=w321) -> (unsigned 16bit integer=w315:u16)
          n187 = To Unsigned Word Integer(number=w323) -> (unsigned 16bit integer=w316:u16)
          n188 = To Unsigned Word Integer(number=w326) -> (unsigned 16bit integer=w317:u16)
          n189 = Add(x="Laser_T", y="Laser_Tshutter") -> (x+y=w310:u16)
          n190 = Replace Array Subset(array=w307, new element=w304, index=w305) -> (w306:u16[])
          n191 = Replace Array Subset(array=w309, new element #1=w328, index #1=w295, new element #2="Laser_Freq", index #2=w296, new element #3="Laser_T", index #3=w297, new element #4="Laser_Tpeak", index #4=w298, new element #5="Laser_Tshutter", index #5=w299, new element #6=w315, index #6=w300, new element #7=w316, index #7=w301, new element #8=w317, index #8=w302, new element #9=w310, index #9=w303) -> (w308:u16[])
        }
        frame 6 {
          n192 = call "BRig_dataExp_L_freq_l2.vi"() -> ("output_L_freq_l2"=w331:i32)  [unwired: 11 in]
          n193 = call "BRig_dataExp_L_T_l2.vi"() -> ("output_L_T_l2"=w332:i32)  [unwired: 11 in]
          n194 = call "BRig_dataExp_L_Tpeak_l2.vi"() -> ("output_L_Tpeak_l2"=w333:i32)  [unwired: 11 in]
          n195 = call "BRig_dataExp_L_Tshutter_l2.vi"() -> ("output_L_Tshutter_l2"=w334:i32)  [unwired: 11 in]
          n196 = Replace Array Subset(array=w338, new element=w335, index=w336) -> (w337:u16[])
          n197 = call "BRig_RT__Case_Idle__calc_LaserPulse.vi"("input_dataExp_L_Tshutter"=w334, "input_dataExp_L_Tpeak"=w333, "input_dataExp_L_T"=w332, "input_dataExp_L_freq"=w331, "input_dataExp"=w340) -> ("output_cluster"=→"LaserPulseTrain":cluster{u16[], u16[]})  [unwired: 6 in]
        }
      }
    }
    frame True {
      w497 = 100.0 ("y")
      n198 = call "BRig_dataLC_ENL_First_OnOff_l2.vi"() -> ("output_ENL_First_OnOff_l2"=w429:i32)  [unwired: 11 in]
      n199 = call "BRig_dataLC_ENL_First_Block_l2.vi"() -> ("output_ENL_First_Block_l2"=w428:i32)  [unwired: 11 in]
      n200 = call "BRig_dataLC_ENL_First_Prob_l2.vi"() -> ("output_ENL_First_Prob_l2"=w430:i32)  [unwired: 11 in]
      n201 = call "BRig_dataLC_ENL_First_Delay_l2.vi"() -> ("output_ENL_First_Delay_l2"=w431:i32)  [unwired: 11 in]
      n202 = call "BRig_dataLC_ENL_First_DelayOpt_l2.vi"() -> ("output_ENL_First_DelayOpt_l2"=w432:i32)  [unwired: 11 in]
      n203 = call "BRig_dataLC_ENL_First_Count_l2.vi"() -> ("output_ENL_First_Count_l2"=w433:i32)  [unwired: 11 in]
      n204 = call "BRig_dataLC_ENL_PreR_OnOff_l2.vi"() -> ("output_ENL_PreR_OnOff_l2"=w434:i32)  [unwired: 11 in]
      n205 = call "BRig_dataLC_ENL_PreR_Block_l2.vi"() -> ("output_ENL_PreR_Block_l2"=w435:i32)  [unwired: 11 in]
      n206 = call "BRig_dataLC_ENL_PreR_Prob_l2.vi"() -> ("output_ENL_PreR_Prob_l2"=w436:i32)  [unwired: 11 in]
      n207 = call "BRig_dataLC_ENL_PreR_Delay_l2.vi"() -> ("output_ENL_PreR_Delay_l2"=w437:i32)  [unwired: 11 in]
      n208 = call "BRig_dataLC_ENL_PreR_DelayOpt_l2.vi"() -> ("output_ENL_PreR_DelayOpt_l2"=w438:i32)  [unwired: 11 in]
      n209 = call "BRig_dataLC_ENL_PreR_Count_l2.vi"() -> ("output_ENL_PreR_Count_l2"=w439:i32)  [unwired: 11 in]
      n210 = call "BRig_dataLC_ENL_PostR_OnOff_l2.vi"() -> ("output_ENL_PostR_OnOff_l2"=w440:i32)  [unwired: 11 in]
      n211 = call "BRig_dataLC_ENL_PostR_Block_l2.vi"() -> ("output_ENL_PostR_Block_l2"=w441:i32)  [unwired: 11 in]
      n212 = call "BRig_dataLC_ENL_PostR_Prob_l2.vi"() -> ("output_ENL_PostR_Prob_l2"=w442:i32)  [unwired: 11 in]
      n213 = call "BRig_dataLC_ENL_PostR_Delay_l2.vi"() -> ("output_ENL_PostR_Delay_l2"=w443:i32)  [unwired: 11 in]
      n214 = call "BRig_dataLC_ENL_PostR_DelayOpt_l2.vi"() -> ("output_ENL_PostR_DelayOpt_l2"=w444:i32)  [unwired: 11 in]
      n215 = call "BRig_dataLC_ENL_PostR_Count_l2.vi"() -> ("output_ENL_PostR_Count_l2"=w445:i32)  [unwired: 11 in]
      n216 = call "BRig_dataLC_ENL2_First_OnOff_l2.vi"() -> ("output_ENL2_First_OnOff_l2"=w364:i32)  [unwired: 11 in]
      n217 = call "BRig_dataLC_ENL2_First_Block_l2.vi"() -> ("output_ENL2_First_Block_l2"=w363:i32)  [unwired: 11 in]
      n218 = call "BRig_dataLC_ENL2_First_Prob_l2.vi"() -> ("output_ENL2_First_Prob_l2"=w362:i32)  [unwired: 11 in]
      n219 = call "BRig_dataLC_ENL2_First_Delay_l2.vi"() -> ("output_ENL2_First_Delay_l2"=w361:i32)  [unwired: 11 in]
      n220 = call "BRig_dataLC_ENL2_First_DelayOpt_l2.vi"() -> ("output_ENL2_First_DelayOpt_l2"=w360:i32)  [unwired: 11 in]
      n221 = call "BRig_dataLC_ENL2_First_Count_l2.vi"() -> ("output_ENL2_First_Count_l2"=w359:i32)  [unwired: 11 in]
      n222 = call "BRig_dataLC_ENL2_PreR_OnOff_l2.vi"() -> ("output_ENL2_PreR_OnOff_l2"=w370:i32)  [unwired: 11 in]
      n223 = call "BRig_dataLC_ENL2_PreR_Block_l2.vi"() -> ("output_ENL2_PreR_Block_l2"=w369:i32)  [unwired: 11 in]
      n224 = call "BRig_dataLC_ENL2_PreR_Prob_l2.vi"() -> ("output_ENL2_PreR_Prob_l2"=w368:i32)  [unwired: 11 in]
      n225 = call "BRig_dataLC_ENL2_PreR_Delay_l2.vi"() -> ("output_ENL2_PreR_Delay_l2"=w367:i32)  [unwired: 11 in]
      n226 = call "BRig_dataLC_ENL2_PreR_DelayOpt_l2.vi"() -> ("output_ENL2_PreR_DelayOpt_l2"=w366:i32)  [unwired: 11 in]
      n227 = call "BRig_dataLC_ENL2_PreR_Count_l2.vi"() -> ("output_ENL2_PreR_Count_l2"=w365:i32)  [unwired: 11 in]
      n228 = call "BRig_dataLC_ENL2_PostR_OnOff_l2.vi"() -> ("output_ENL2_PostR_OnOff_l2"=w376:i32)  [unwired: 11 in]
      n229 = call "BRig_dataLC_ENL2_PostR_Block_l2.vi"() -> ("output_ENL2_PostR_Block_l2"=w375:i32)  [unwired: 11 in]
      n230 = call "BRig_dataLC_ENL2_PostR_Prob_l2.vi"() -> ("output_ENL2_PostR_Prob_l2"=w374:i32)  [unwired: 11 in]
      n231 = call "BRig_dataLC_ENL2_PostR_Delay_l2.vi"() -> ("output_ENL2_PostR_Delay_l2"=w373:i32)  [unwired: 11 in]
      n232 = call "BRig_dataLC_ENL2_PostR_DelayOpt_l2.vi"() -> ("output_ENL2_PostR_DelayOpt_l2"=w372:i32)  [unwired: 11 in]
      n233 = call "BRig_dataLC_ENL2_PostR_Count_l2.vi"() -> ("output_ENL2_PostR_Count_l2"=w371:i32)  [unwired: 11 in]
      n234 = Index Array(array=w511, index #1=w429, index #2=w428, index #3=w430, index #4=w431, index #5=w432, index #6=w433, index #7=w434, index #8=w435, index #9=w436, index #10=w437, index #11=w438, index #12=w439, index #13=w440, index #14=w441, index #15=w442, index #16=w443, index #17=w444, index #18=w445) -> (element #1=w583:u16, element #2=w582:u16, element #3=w581:u16, element #4=w580:u16, element #5=w579:u16, element #6=w578:u16, element #7=w577:u16, element #8=w576:u16, element #9=w575:u16, element #10=w574:u16, element #11=w573:u16, element #12=w572:u16, element #13=w571:u16, element #14=w570:u16, element #15=w569:u16, element #16=w568:u16, element #17=w567:u16, element #18=w566:u16)
      n235 = Index Array(array=w464, index #1=w364, index #2=w363, index #3=w362, index #4=w361, index #5=w360, index #6=w359, index #7=w370, index #8=w369, index #9=w368, index #10=w367, index #11=w366, index #12=w365, index #13=w376, index #14=w375, index #15=w374, index #16=w373, index #17=w372, index #18=w371) -> (element #1=w471:u16, element #2=w472:u16, element #3=w473:u16, element #4=w474:u16, element #5=w475:u16, element #6=w476:u16, element #7=w477:u16, element #8=w478:u16, element #9=w479:u16, element #10=w480:u16, element #11=w481:u16, element #12=w482:u16, element #13=w484:u16, element #14=w485:u16, element #15=w486:u16, element #16=w487:u16, element #17=w488:u16, element #18=w489:u16)
      n236 = Not Equal To 0?(x=w583) -> (x != 0?=w589:bool)
      n237 = Not Equal To 0?(x=w579) -> (x != 0?=w588:bool)
      n238 = Not Equal To 0?(x=w577) -> (x != 0?=w587:bool)
      n239 = Not Equal To 0?(x=w573) -> (x != 0?=w586:bool)
      n240 = Not Equal To 0?(x=w571) -> (x != 0?=w585:bool)
      n241 = Not Equal To 0?(x=w567) -> (x != 0?=w584:bool)
      n242 = local write "LC_ENL_First_OnOff"(w589) -> ()
      n243 = local write "LC_ENL_First_Block"(w582) -> ()
      n244 = local write "LC_ENL_First_Probability"(w581) -> ()
      n245 = local write "LC_ENL_First_Tdelay"(w580) -> ()
      n246 = local write "LC_ENL_First_delayOpt"(w588) -> ()
      n247 = local write "LC_ENL_First_Count"(w578) -> ()
      n248 = local write "LC_ENL_PreR_OnOff"(w587) -> ()
      n249 = local write "LC_ENL_PreR_Block"(w576) -> ()
      n250 = local write "LC_ENL_PreR_Probability"(w575) -> ()
      n251 = local write "LC_ENL_PreR_Tdelay"(w574) -> ()
      n252 = local write "LC_ENL_PreR_delayOpt"(w586) -> ()
      n253 = local write "LC_ENL_PreR_Count"(w572) -> ()
      n254 = local write "LC_ENL_PostR_OnOff"(w585) -> ()
      n255 = local write "LC_ENL_PostR_Block"(w570) -> ()
      n256 = local write "LC_ENL_PostR_Probability"(w569) -> ()
      n257 = local write "LC_ENL_PostR_Tdelay"(w568) -> ()
      n258 = local write "LC_ENL_PostR_delayOpt"(w584) -> ()
      n259 = local write "LC_ENL_PostR_Count"(w566) -> ()
      n260 = Not Equal To 0?(x=w471) -> (x != 0?=w492:bool)
      n261 = Not Equal To 0?(x=w475) -> (x != 0?=w493:bool)
      n262 = Not Equal To 0?(x=w477) -> (x != 0?=w491:bool)
      n263 = Not Equal To 0?(x=w481) -> (x != 0?=w494:bool)
      n264 = Not Equal To 0?(x=w484) -> (x != 0?=w490:bool)
      n265 = Not Equal To 0?(x=w488) -> (x != 0?=w483:bool)
      n266 = local write "LC_ENL2_First_OnOff"(w492) -> ()
      n267 = local write "LC_ENL2_First_Block"(w472) -> ()
      n268 = local write "LC_ENL2_First_Probability"(w473) -> ()
      n269 = local write "LC_ENL2_First_Tdelay"(w474) -> ()
      n270 = local write "LC_ENL2_First_delayOpt"(w493) -> ()
      n271 = local write "LC_ENL2_First_Count"(w476) -> ()
      n272 = local write "LC_ENL2_PreR_OnOff"(w491) -> ()
      n273 = local write "LC_ENL2_PreR_Block"(w478) -> ()
      n274 = local write "LC_ENL2_PreR_Probability"(w479) -> ()
      n275 = local write "LC_ENL2_PreR_Tdelay"(w480) -> ()
      n276 = local write "LC_ENL2_PreR_delayOpt"(w494) -> ()
      n277 = local write "LC_ENL2_PreR_Count"(w482) -> ()
      n278 = local write "LC_ENL2_PostR_OnOff"(w490) -> ()
      n279 = local write "LC_ENL2_PostR_Block"(w485) -> ()
      n280 = local write "LC_ENL2_PostR_Probability"(w486) -> ()
      n281 = local write "LC_ENL2_PostR_Tdelay"(w487) -> ()
      n282 = local write "LC_ENL2_PostR_delayOpt"(w483) -> ()
      n283 = local write "LC_ENL2_PostR_Count"(w489) -> ()
      n284 = call "BRig_dataLC_Cue_First_OnOff_l2.vi"() -> ("output_Cue_First_OnOff_l2"=w412:i32)  [unwired: 11 in]
      n285 = call "BRig_dataLC_Cue_First_Block_l2.vi"() -> ("output_Cue_First_Block_l2"=w410:i32)  [unwired: 11 in]
      n286 = call "BRig_dataLC_Cue_First_Prob_l2.vi"() -> ("output_Cue_First_Prob_l2"=w411:i32)  [unwired: 11 in]
      n287 = call "BRig_dataLC_Cue_First_Delay_l2.vi"() -> ("output_Cue_First_Delay_l2"=w413:i32)  [unwired: 11 in]
      n288 = call "BRig_dataLC_Cue_First_DelayOpt_l2.vi"() -> ("output_Cue_First_DelayOpt_l2"=w414:i32)  [unwired: 11 in]
      n289 = call "BRig_dataLC_Cue_First_Count_l2.vi"() -> ("output_Cue_First_Count_l2"=w415:i32)  [unwired: 11 in]
      n290 = call "BRig_dataLC_Cue_PreR_OnOff_l2.vi"() -> ("output_Cue_PreR_OnOff_l2"=w416:i32)  [unwired: 11 in]
      n291 = call "BRig_dataLC_Cue_PreR_Block_l2.vi"() -> ("output_Cue_PreR_Block_l2"=w417:i32)  [unwired: 11 in]
      n292 = call "BRig_dataLC_Cue_PreR_Prob_l2.vi"() -> ("output_Cue_PreR_Prob_l2"=w418:i32)  [unwired: 11 in]
      n293 = call "BRig_dataLC_Cue_PreR_Delay_l2.vi"() -> ("output_Cue_PreR_Delay_l2"=w419:i32)  [unwired: 11 in]
      n294 = call "BRig_dataLC_Cue_PreR_DelayOpt_l2.vi"() -> ("output_Cue_PreR_DelayOpt_l2"=w420:i32)  [unwired: 11 in]
      n295 = call "BRig_dataLC_Cue_PreR_Count_l2.vi"() -> ("output_Cue_PreR_Count_l2"=w421:i32)  [unwired: 11 in]
      n296 = call "BRig_dataLC_Cue_PostR_OnOff_l2.vi"() -> ("output_Cue_PostR_OnOff_l2"=w422:i32)  [unwired: 11 in]
      n297 = call "BRig_dataLC_Cue_PostR_Block_l2.vi"() -> ("output_Cue_PostR_Block_l2"=w423:i32)  [unwired: 11 in]
      n298 = call "BRig_dataLC_Cue_PostR_Prob_l2.vi"() -> ("output_Cue_PostR_Prob_l2"=w424:i32)  [unwired: 11 in]
      n299 = call "BRig_dataLC_Cue_PostR_Delay_l2.vi"() -> ("output_Cue_PostR_Delay_l2"=w425:i32)  [unwired: 11 in]
      n300 = call "BRig_dataLC_Cue_PostR_DelayOpt_l2.vi"() -> ("output_Cue_PostR_DelayOpt_l2"=w426:i32)  [unwired: 11 in]
      n301 = call "BRig_dataLC_Cue_PostR_Count_l2.vi"() -> ("output_Cue_PostR_Count_l2"=w427:i32)  [unwired: 11 in]
      n302 = call "BRig_dataExp_LED_baseline_l2.vi"() -> ("output_LED_baseline_l2"=w384:i32)  [unwired: 11 in]
      n303 = call "BRig_dataExp_L_freq_l2.vi"() -> ("output_L_freq_l2"=w383:i32)  [unwired: 11 in]
      n304 = call "BRig_dataExp_L_T_l2.vi"() -> ("output_L_T_l2"=w382:i32)  [unwired: 11 in]
      n305 = call "BRig_dataExp_L_Tpeak_l2.vi"() -> ("output_L_Tpeak_l2"=w381:i32)  [unwired: 11 in]
      n306 = call "BRig_dataExp_L_Tshutter_l2.vi"() -> ("output_L_Tshutter_l2"=w380:i32)  [unwired: 11 in]
      n307 = call "BRig_dataExp_L_power_min_l2.vi"() -> ("output_L_power_min_l2"=w379:i32)  [unwired: 11 in]
      n308 = call "BRig_dataExp_L_power_max_l2.vi"() -> ("output_L_power_max_l2"=w378:i32)  [unwired: 11 in]
      n309 = call "BRig_dataExp_L_power_step_l2.vi"() -> ("output_L_power_step_l2"=w377:i32)  [unwired: 11 in]
      n310 = Index Array(array=w511, index #1=w412, index #2=w410, index #3=w411, index #4=w413, index #5=w414, index #6=w415, index #7=w416, index #8=w417, index #9=w418, index #10=w419, index #11=w420, index #12=w421, index #13=w422, index #14=w423, index #15=w424, index #16=w425, index #17=w426, index #18=w427) -> (element #1=w559:u16, element #2=w558:u16, element #3=w557:u16, element #4=w556:u16, element #5=w555:u16, element #6=w554:u16, element #7=w553:u16, element #8=w552:u16, element #9=w551:u16, element #10=w550:u16, element #11=w549:u16, element #12=w548:u16, element #13=w547:u16, element #14=w546:u16, element #15=w545:u16, element #16=w544:u16, element #17=w543:u16, element #18=w542:u16)
      n311 = Index Array(array=w464, index #1=w384, index #2=w383, index #3=w382, index #4=w381, index #5=w380, index #6=w379, index #7=w378, index #8=w377) -> (element #1=w510:u16, element #2=w508:u16, element #3=w507:u16, element #4=w506:u16, element #5=w505:u16, element #6=w504:u16, element #7=w503:u16, element #8=w502:u16)
      n312 = To Double Precision Float(number=w504) -> (double precision float=w501:dbl)
      n313 = To Double Precision Float(number=w503) -> (double precision float=w496:dbl)
      n314 = To Double Precision Float(number=w502) -> (double precision float=w495:dbl)
      n315 = Not Equal To 0?(x=w559) -> (x != 0?=w565:bool)
      n316 = Not Equal To 0?(x=w555) -> (x != 0?=w564:bool)
      n317 = Not Equal To 0?(x=w553) -> (x != 0?=w563:bool)
      n318 = Not Equal To 0?(x=w549) -> (x != 0?=w562:bool)
      n319 = Not Equal To 0?(x=w547) -> (x != 0?=w561:bool)
      n320 = Not Equal To 0?(x=w543) -> (x != 0?=w560:bool)
      n321 = Divide(x=w501, y=w497) -> (x/y=w500:dbl)
      n322 = Divide(x=w496, y=w497) -> (x/y=w499:dbl)
      n323 = Divide(x=w495, y=w497) -> (x/y=w498:dbl)
      n324 = local write "LC_Cue_First_OnOff"(w565) -> ()
      n325 = local write "LC_Cue_First_Block"(w558) -> ()
      n326 = local write "LC_Cue_First_Probability"(w557) -> ()
      n327 = local write "LC_Cue_First_Tdelay"(w556) -> ()
      n328 = local write "LC_Cue_First_delayOpt"(w564) -> ()
      n329 = local write "LC_Cue_First_Count"(w554) -> ()
      n330 = local write "LC_Cue_PreR_OnOff"(w563) -> ()
      n331 = local write "LC_Cue_PreR_Block"(w552) -> ()
      n332 = local write "LC_Cue_PreR_Probability"(w551) -> ()
      n333 = local write "LC_Cue_PreR_Tdelay"(w550) -> ()
      n334 = local write "LC_Cue_PreR_delayOpt"(w562) -> ()
      n335 = local write "LC_Cue_PreR_Count"(w548) -> ()
      n336 = local write "LC_Cue_PostR_OnOff"(w561) -> ()
      n337 = local write "LC_Cue_PostR_Block"(w546) -> ()
      n338 = local write "LC_Cue_PostR_Probability"(w545) -> ()
      n339 = local write "LC_Cue_PostR_Tdelay"(w544) -> ()
      n340 = local write "LC_Cue_PostR_delayOpt"(w560) -> ()
      n341 = local write "LC_Cue_PostR_Count"(w542) -> ()
      n342 = Not Equal To 0?(x=w510) -> (x != 0?=w509:bool)
      n343 = call "BRig_dataLC_Cue2_First_OnOff_l2.vi"() -> ("output_Cue2_First_OnOff_l2"=w358:i32)  [unwired: 11 in]
      n344 = call "BRig_dataLC_Cue2_First_Block_l2.vi"() -> ("output_Cue2_First_Block_l2"=w357:i32)  [unwired: 11 in]
      n345 = call "BRig_dataLC_Cue2_First_Prob_l2.vi"() -> ("output_Cue2_First_Prob_l2"=w356:i32)  [unwired: 11 in]
      n346 = call "BRig_dataLC_Cue2_First_Delay_l2.vi"() -> ("output_Cue2_First_Delay_l2"=w355:i32)  [unwired: 11 in]
      n347 = call "BRig_dataLC_Cue2_First_DelayOpt_l2.vi"() -> ("output_Cue2_First_DelayOpt_l2"=w354:i32)  [unwired: 11 in]
      n348 = call "BRig_dataLC_Cue2_First_Count_l2.vi"() -> ("output_Cue2_First_Count_l2"=w353:i32)  [unwired: 11 in]
      n349 = call "BRig_dataLC_Cue2_PostR_OnOff_l2.vi"() -> ("output_Cue2_PostR_OnOff_l2"=w352:i32)  [unwired: 11 in]
      n350 = call "BRig_dataLC_Cue2_PostR_Block_l2.vi"() -> ("output_Cue2_PostR_Block_l2"=w351:i32)  [unwired: 11 in]
      n351 = call "BRig_dataLC_Cue2_PostR_Prob_l2.vi"() -> ("output_Cue2_PostR_Prob_l2"=w350:i32)  [unwired: 11 in]
      n352 = call "BRig_dataLC_Cue2_PostR_Delay_l2.vi"() -> ("output_Cue2_PostR_Delay_l2"=w349:i32)  [unwired: 11 in]
      n353 = call "BRig_dataLC_Cue2_PostR_DelayOpt_l2.vi"() -> ("output_Cue2_PostR_DelayOpt_l2"=w348:i32)  [unwired: 11 in]
      n354 = call "BRig_dataLC_Cue2_PostR_Count_l2.vi"() -> ("output_Cue2_PostR_Count_l2"=w347:i32)  [unwired: 11 in]
      n355 = call "BRig_dataLC_Cue2_PreR_OnOff_l2.vi"() -> ("output_Cue2_PreR_OnOff_l2"=w346:i32)  [unwired: 11 in]
      n356 = call "BRig_dataLC_Cue2_PreR_Block_l2.vi"() -> ("output_Cue2_PreR_Block_l2"=w345:i32)  [unwired: 11 in]
      n357 = call "BRig_dataLC_Cue2_PreR_Prob_l2.vi"() -> ("output_Cue2_PreR_Prob_l2"=w344:i32)  [unwired: 11 in]
      n358 = call "BRig_dataLC_Cue2_PreR_Delay_l2.vi"() -> ("output_Cue2_PreR_Delay_l2"=w343:i32)  [unwired: 11 in]
      n359 = call "BRig_dataLC_Cue2_PreR_DelayOpt_l2.vi"() -> ("output_Cue2_PreR_DelayOpt_l2"=w342:i32)  [unwired: 11 in]
      n360 = call "BRig_dataLC_Cue2_PreR_Count_l2.vi"() -> ("output_Cue2_PreR_Count_l2"=w341:i32)  [unwired: 11 in]
      n361 = local write "LED_baseline"(w509) -> ()
      n362 = local write "Laser_Freq"(w508) -> ()
      n363 = local write "Laser_T"(w507) -> ()
      n364 = local write "Laser_Tpeak"(w506) -> ()
      n365 = local write "Laser_Tshutter"(w505) -> ()
      n366 = local write "Laser_power_min"(w500) -> ()
      n367 = local write "Laser_power_max"(w499) -> ()
      n368 = local write "Laser_power_step"(w498) -> ()
      n369 = Index Array(array=w464, index #1=w358, index #2=w357, index #3=w356, index #4=w355, index #5=w354, index #6=w353, index #7=w352, index #8=w351, index #9=w350, index #10=w349, index #11=w348, index #12=w347, index #13=w346, index #14=w345, index #15=w344, index #16=w343, index #17=w342, index #18=w341) -> (element #1=w465:u16, element #2=w460:u16, element #3=w459:u16, element #4=w458:u16, element #5=w466:u16, element #6=w461:u16, element #7=w467:u16, element #8=w455:u16, element #9=w454:u16, element #10=w453:u16, element #11=w468:u16, element #12=w452:u16, element #13=w469:u16, element #14=w449:u16, element #15=w448:u16, element #16=w447:u16, element #17=w470:u16, element #18=w446:u16)
      n370 = call "BRig_dataLC_Selection_First_OnOff_l2.vi"() -> ("output_Selection_First_OnOff_l2"=w409:i32)  [unwired: 11 in]
      n371 = call "BRig_dataLC_Selection_First_Block_l2.vi"() -> ("output_Selection_First_Block_l2"=w408:i32)  [unwired: 11 in]
      n372 = call "BRig_dataLC_Selection_First_Prob_l2.vi"() -> ("output_Selection_First_Prob_l2"=w407:i32)  [unwired: 11 in]
      n373 = call "BRig_dataLC_Selection_First_Delay_l2.vi"() -> ("output_Selection_First_Delay_l2"=w406:i32)  [unwired: 11 in]
      n374 = call "BRig_dataLC_Selection_First_Count_l2.vi"() -> ("output_Selection_First_Count_l2"=w405:i32)  [unwired: 11 in]
      n375 = call "BRig_dataLC_Selection_PreR_OnOff_l2.vi"() -> ("output_Selection_PreR_OnOff_l2"=w404:i32)  [unwired: 11 in]
      n376 = call "BRig_dataLC_Selection_PreR_Block_l2.vi"() -> ("output_Selection_PreR_Block_l2"=w403:i32)  [unwired: 11 in]
      n377 = call "BRig_dataLC_Selection_PreR_Prob_l2.vi"() -> ("output_Selection_PreR_Prob_l2"=w402:i32)  [unwired: 11 in]
      n378 = call "BRig_dataLC_Selection_PreR_Delay_l2.vi"() -> ("output_Selection_PreR_Delay_l2"=w401:i32)  [unwired: 11 in]
      n379 = call "BRig_dataLC_Selection_PreR_Count_l2.vi"() -> ("output_Selection_PreR_Count_l2"=w400:i32)  [unwired: 11 in]
      n380 = call "BRig_dataLC_Selection_PostR_OnOff_l2.vi"() -> ("output_Selection_PostR_OnOff_l2"=w399:i32)  [unwired: 11 in]
      n381 = call "BRig_dataLC_Selection_PostR_Block_l2.vi"() -> ("output_Selection_PostR_Block_l2"=w398:i32)  [unwired: 11 in]
      n382 = call "BRig_dataLC_Selection_PostR_Prob_l2.vi"() -> ("output_Selection_PostR_Prob_l2"=w397:i32)  [unwired: 11 in]
      n383 = call "BRig_dataLC_Selection_PostR_Delay_l2.vi"() -> ("output_Selection_PostR_Delay_l2"=w396:i32)  [unwired: 11 in]
      n384 = call "BRig_dataLC_Selection_PostR_Count_l2.vi"() -> ("output_Selection_PostR_Count_l2"=w395:i32)  [unwired: 11 in]
      n385 = call "BRig_dataLC_Reward_OnOff_l2.vi"() -> ("output_Reward_OnOff_l2"=w385:i32)  [unwired: 11 in]
      n386 = call "BRig_dataLC_Reward_Block_l2.vi"() -> ("output_Reward_Block_l2"=w386:i32)  [unwired: 11 in]
      n387 = call "BRig_dataLC_Reward_Trial_l2.vi"() -> ("output_Reward_Trial_l2"=w387:i32)  [unwired: 11 in]
      n388 = call "BRig_dataLC_Reward_Prob_l2.vi"() -> ("output_Reward_Prob_l2"=w388:i32)  [unwired: 11 in]
      n389 = call "BRig_dataLC_Reward_Delay_l2.vi"() -> ("output_Reward_Delay_l2"=w389:i32)  [unwired: 11 in]
      n390 = call "BRig_dataLC_Wrong_OnOff_l2.vi"() -> ("output_Wrong_OnOff_l2"=w390:i32)  [unwired: 11 in]
      n391 = call "BRig_dataLC_Wrong_Block_l2.vi"() -> ("output_Wrong_Block_l2"=w391:i32)  [unwired: 11 in]
      n392 = call "BRig_dataLC_Wrong_Trial_l2.vi"() -> ("output_Wrong_Trial_l2"=w392:i32)  [unwired: 11 in]
      n393 = call "BRig_dataLC_Wrong_Prob_l2.vi"() -> ("output_Wrong_Prob_l2"=w393:i32)  [unwired: 11 in]
      n394 = call "BRig_dataLC_Wrong_Delay_l2.vi"() -> ("output_Wrong_Delay_l2"=w394:i32)  [unwired: 11 in]
      n395 = Not Equal To 0?(x=w465) -> (x != 0?=w463:bool)
      n396 = Not Equal To 0?(x=w466) -> (x != 0?=w462:bool)
      n397 = Not Equal To 0?(x=w467) -> (x != 0?=w456:bool)
      n398 = Not Equal To 0?(x=w468) -> (x != 0?=w457:bool)
      n399 = Not Equal To 0?(x=w469) -> (x != 0?=w451:bool)
      n400 = Not Equal To 0?(x=w470) -> (x != 0?=w450:bool)
      n401 = Index Array(array=w511, index #1=w385, index #2=w386, index #3=w387, index #4=w388, index #5=w389, index #6=w390, index #7=w391, index #8=w392, index #9=w393, index #10=w394) -> (element #1=w521:u16, element #2=w520:u16, element #3=w519:u16, element #4=w518:u16, element #5=w517:u16, element #6=w516:u16, element #7=w515:u16, element #8=w514:u16, element #9=w513:u16, element #10=w512:u16)
      n402 = local write "LC_Cue2_First_OnOff"(w463) -> ()
      n403 = local write "LC_Cue2_First_Block"(w460) -> ()
      n404 = local write "LC_Cue2_First_Probability"(w459) -> ()
      n405 = local write "LC_Cue2_First_Tdelay"(w458) -> ()
      n406 = local write "LC_Cue2_First_delayOpt"(w462) -> ()
      n407 = local write "LC_Cue2_First_Count"(w461) -> ()
      n408 = local write "LC_Cue2_PreR_OnOff"(w456) -> ()
      n409 = local write "LC_Cue2_PreR_Block"(w455) -> ()
      n410 = local write "LC_Cue2_PreR_Probability"(w454) -> ()
      n411 = local write "LC_Cue2_PreR_Tdelay"(w453) -> ()
      n412 = local write "LC_Cue2_PreR_delayOpt"(w457) -> ()
      n413 = local write "LC_Cue2_PreR_Count"(w452) -> ()
      n414 = local write "LC_Cue2_PostR_OnOff"(w451) -> ()
      n415 = local write "LC_Cue2_PostR_Block"(w449) -> ()
      n416 = local write "LC_Cue2_PostR_Probability"(w448) -> ()
      n417 = local write "LC_Cue2_PostR_Tdelay"(w447) -> ()
      n418 = local write "LC_Cue2_PostR_delayOpt"(w450) -> ()
      n419 = local write "LC_Cue2_PostR_Count"(w446) -> ()
      n420 = Index Array(array=w511, index #1=w409, index #2=w408, index #3=w407, index #4=w406, index #5=w405, index #6=w404, index #7=w403, index #8=w402, index #9=w401, index #10=w400, index #11=w399, index #12=w398, index #13=w397, index #14=w396, index #15=w395) -> (element #1=w538:u16, element #2=w537:u16, element #3=w536:u16, element #4=w535:u16, element #5=w534:u16, element #6=w533:u16, element #7=w532:u16, element #8=w531:u16, element #9=w530:u16, element #10=w529:u16, element #11=w528:u16, element #12=w527:u16, element #13=w526:u16, element #14=w525:u16, element #15=w524:u16)
      n421 = Not Equal To 0?(x=w521) -> (x != 0?=w523:bool)
      n422 = Not Equal To 0?(x=w516) -> (x != 0?=w522:bool)
      n423 = Not Equal To 0?(x=w538) -> (x != 0?=w541:bool)
      n424 = Not Equal To 0?(x=w533) -> (x != 0?=w540:bool)
      n425 = Not Equal To 0?(x=w528) -> (x != 0?=w539:bool)
      n426 = local write "LC_Reward_OnOff"(w523) -> ()
      n427 = local write "LC_Reward_Block"(w520) -> ()
      n428 = local write "LC_Reward_Trial"(w519) -> ()
      n429 = local write "LC_Reward_Probability"(w518) -> ()
      n430 = local write "LC_Reward_Tdelay"(w517) -> ()
      n431 = local write "LC_Wrong_OnOff"(w522) -> ()
      n432 = local write "LC_Wrong_Block"(w515) -> ()
      n433 = local write "LC_Wrong_Trial"(w514) -> ()
      n434 = local write "LC_Wrong_Probability"(w513) -> ()
      n435 = local write "LC_Wrong_Tdelay"(w512) -> ()
      n436 = local write "LC_Sel_First_OnOff"(w541) -> ()
      n437 = local write "LC_Sel_First_Block"(w537) -> ()
      n438 = local write "LC_Sel_First_Probability"(w536) -> ()
      n439 = local write "LC_Sel_First_Tdelay"(w535) -> ()
      n440 = local write "LC_Sel_First_Count"(w534) -> ()
      n441 = local write "LC_Sel_PreR_OnOff"(w540) -> ()
      n442 = local write "LC_Sel_PreR_Block"(w532) -> ()
      n443 = local write "LC_Sel_PreR_Probability"(w531) -> ()
      n444 = local write "LC_Sel_PreR_Tdelay"(w530) -> ()
      n445 = local write "LC_Sel_PreR_Count"(w529) -> ()
      n446 = local write "LC_Sel_PostR_OnOff"(w539) -> ()
      n447 = local write "LC_Sel_PostR_Block"(w527) -> ()
      n448 = local write "LC_Sel_PostR_Probability"(w526) -> ()
      n449 = local write "LC_Sel_PostR_Tdelay"(w525) -> ()
      n450 = local write "LC_Sel_PostR_Count"(w524) -> ()
    }
  }
  "output_dataLC" <- w4
  "output_dataExp" <- w1
